vi "Saccade-Analyser.vi"(3 "EMA-Data IN":T4={"Impulse Positions"=[], "No. Imp"=0, "Parameter Time Series"=[], "Parameter Impuls Series"=[], "Experiment Parameters"={"Freq"=0.0, "Vel"=0, "Acc"=0, "Stimulus"=""}, "Autosort File"=refnum, "Data File"={"Data Channels"=[], "Sample Rate"=0, "Channel List"=[]}, "Experiment data path"=path "/Macintosh HD/Users/patrick/Studium/Diploma Thesis/Data Analysis", "Image data path"=path "/Macintosh HD/Users/patrick/Studium/Diploma Thesis/Data Analysis", "LVS data path"=path "/Macintosh HD/Users/patrick/Studium/Diploma Thesis/Data Analysis", "Raw copy path"=path "/Macintosh HD/Users/patrick/Studium/Diploma Thesis/Data Analysis", "filename"="No file selected", "desaccading parameters"={"Tolerance"=0, "Acc Range"=0.0, "Sample Rate"=0, "Impulse Plane 2"=enum."Other", "Impulse dir"=FALSE}, "Experiment Parameters 2"={"Subject"="", "Strain"="", "Rotation plane"="", "Experimenter"="", "Trial"=0.0, "Time"=0.0}, "Excel"={"Excel._Application"=refnum, "Use Excel"=FALSE, "Worksheet SINE"=refnum, "Row SINE"=0, "Worksheet TRANS"=refnum, "Row TRANS"=0}, "Session Config File"=refnum, "Autosort Parameter Set"=1, "EMA Version"="", "desacc "={"Threshold 1 [Acc]"=1617.080808080808, "Threshold 2 [% of TH1]"=67, "tolerance"=5, "Search WD "=0.19090909090909092, " always use TH2"=TRUE, "Range"=3.2323232323232323, "Max time"=200.0, "Min time"=20.0, "Velocity Threshold"=67}, "Cycle Nr for Saccades"={"POS"=0, "NEG"=0}, "calibration name"="No file selected"} {"Parameter Time Series"."time offset" format="%.3f"; "Parameter Time Series"."Gain" format="%.1f"; "Parameter Time Series"."Offset" format="%.1f"; "Parameter Time Series"."List 1" items=["Motor-Pos", "Motor-Vel", "Lx Position-in-Head", "Ly Position-in-Head", "Lz Position-in-Head", "Lx Velocity-in-Head", "Ly Velocity-in-Head", "Lz Velocity-in-Head", "Ll Velocity-in-Head", "Lr Velocity-in-Head", "Lx Accel-in-Head", "Ly Accel-in-Head", "Lz Accel-in-Head", "Rx Position-in-Head", "Ry Position-in-Head", "Rz Position-in-Head", "Rx Velocity-in-Head", "Ry Velocity-in-Head", "Rz Velocity-in-Head", "Rl Velocity-in-Head", "Rr Velocity-in-Head", "Rx Accel-in-Head", "Ry Accel-in-Head", "Rz Accel-in-Head", "Global Trigger", "", "", ""]; "Parameter Impuls Series"."Gain" format="%.1f"; "Parameter Impuls Series"."Offset" format="%.1f"}) -> ()   [LabVIEW 2016]
uses:
  core/type-defs/TD_Statemachine-Data.ctl
  core/type-defs/TD_Time Series.ctl
  core/type-defs/TD_Impulse Parameter.ctl
  Saccade-Analyzer-TD.ctl
  <vilib>/Utility/miscctls.llb/LVRowAndColumnTypeDef.ctl
  <vilib>/Analysis/baseanly.llb/Mean (DBL).vi
  <vilib>/Analysis/3filter.llb/Savitzky-Golay Filter (DBL).vi
  <vilib>/Analysis/1siggen.llb/Ramp Pattern by Samples.vi
  comm/comm.lvlib
  comm/impulse/impulse functions.lvlib
  <vilib>/Analysis/NI_AALBase.lvlib
  <vilib>/Analysis/NI_AALPro.lvlib
  <vilib>/Analysis/NI_AAL_SigProc.lvlib
  comm/nan operations/nan operations.lvlib
  core/core.lvlib
panel:
  in  "Undo Button":bool
  in  "Amend":bool
  out "Saccade Velocity":dbl[][](graph)
  out "Saccade Position":dbl[][](graph)
  in  "Direction":bool
  in  "Start":bool
  in  "Channel Velocity":u16(ring)=13 items=["Hz Position-in-Head", "Hz Velocity-in-Head", "Hy Position-in-Head", "Hy Velocity-in-Head", "Hx Position-in-Head", "Hx Velocity-in-Head", "Hl Velocity-in-Head", "Hr Velocity-in-Head", "Lx Position-in-Head", "Ly Position-in-Head", "Lz Position-in-Head", "Lx Velocity-in-Head", "Ly Velocity-in-Head", "Lz Velocity-in-Head", "Ll Velocity-in-Head", "Lr Velocity-in-Head", "Rx Position-in-Head", "Ry Position-in-Head", "Rz Position-in-Head", "Rx Velocity-in-Head", "Ry Velocity-in-Head", "Rz Velocity-in-Head", "Rl Velocity-in-Head", "Rr Velocity-in-Head", "Target on/off", "aux input 1", "aux input 2", " ", "", "", "", "Target Hor", "Target Ver", ""]
  in  "Channel Position":u16(ring)=13 items=["Hz Position-in-Head", "Hz Velocity-in-Head", "Hy Position-in-Head", "Hy Velocity-in-Head", "Hx Position-in-Head", "Hx Velocity-in-Head", "Hl Velocity-in-Head", "Hr Velocity-in-Head", "Lx Position-in-Head", "Ly Position-in-Head", "Lz Position-in-Head", "Lx Velocity-in-Head", "Ly Velocity-in-Head", "Lz Velocity-in-Head", "Ll Velocity-in-Head", "Lr Velocity-in-Head", "Rx Position-in-Head", "Ry Position-in-Head", "Rz Position-in-Head", "Rx Velocity-in-Head", "Ry Velocity-in-Head", "Rz Velocity-in-Head", "Rl Velocity-in-Head", "Rr Velocity-in-Head", "Target on/off", "aux input 1", "aux input 2", " ", "", "", "", "Target Hor", "Target Ver", ""]
  in  "Tab Control":T1(tab)
  out "Main Sequence - Velocity vs Position":T2(graph)
  out "Saccade Duration":dbl[][](graph)
  in  "Copy to Clipboard":bool
  out "Mean Saccade Duration [ms]":dbl format="%0.2f"
  out "Main Sequence - Duration vs Position":T2(graph)
  in  "Adjust":bool
  in  "Skip for Analysis":bool caption="Cancel Button"
  out "Single Saccade Display":T3(graph)
  in  "Skip Forward Button":bool
  in  "Pause Button":bool
  in  "Seek Forward Button":bool
  out "Mean Noise":dbl
  out "SD Noise":dbl
  in  "Copy to Clipboard 2":bool
  in  "Table":string[][](table)
  # "Saccade / Quick-Phase Analyser"
  # "(c) Patrick Huebner 2011"
  # "POS"
  # "NEG"
  # "+/-"
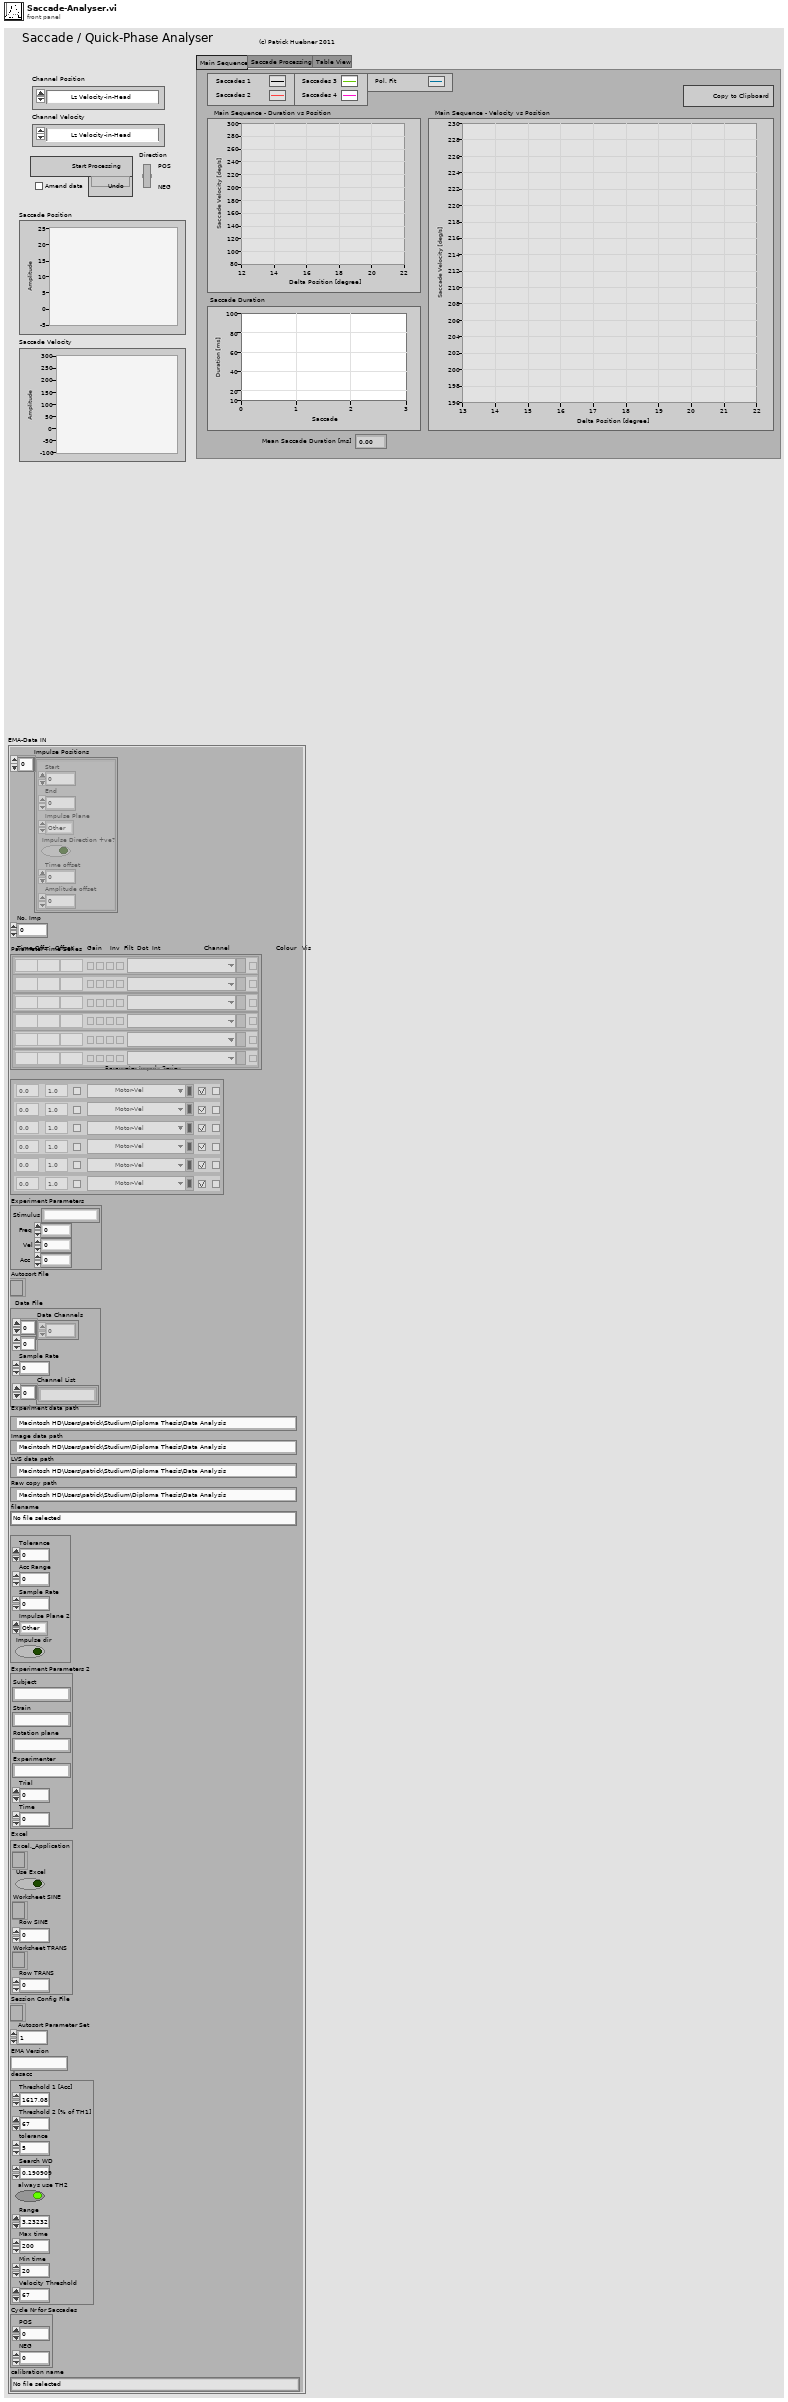
[diagram p1: front panel]
types:
  T1 = enum32{"Main Sequence", "Saccade Processing", "Table View"}
  T2 = cluster{"Best Polynomial Fit":dbl[], "Sorted array":dbl[]}[]
  T3 = cluster{"Ramp Pattern":dbl[], "appended array":dbl[]}[]
  T4 = typedef "core.lvlib/TD_Statemachine-Data.ctl" = cluster{"Impulse Positions":cluster{"Start":i32, "End":i32, "Impulse Plane":enum16{"Other", "Yaw", "Pitch", "Roll", "LARP", "RALP"}, "Impulse Direction +ve?":bool, "Time offset":i32, "Amplitude offset":dbl}[], "No. Imp":i32, "Parameter Time Series":T5, "Parameter Impuls Series":T6, "Experiment Parameters":cluster{"Freq":dbl, "Vel":i32, "Acc":i32, "Stimulus":string}, "Autosort File":refnum<file>, "Data File":cluster{"Data Channels":dbl[][], "Sample Rate":i32, "Channel List":string[]}, "Experiment data path":path, "Image data path":path, "LVS data path":path, "Raw copy path":path, "filename":string, "desaccading parameters":cluster{"Tolerance":i32, "Acc Range":dbl, "Sample Rate":i32, "Impulse Plane 2":enum16{"Other", "Yaw", "Pitch", "Roll", "LARP", "RALP"}, "Impulse dir":bool}, "Experiment Parameters 2":cluster{"Subject":string, "Strain":string, "Rotation plane":string, "Experimenter":string, "Trial":dbl, "Time":dbl}, "Excel":cluster{"Excel._Application":refnum<k7>, "Use Excel":bool, "Worksheet SINE":refnum<k7>, "Row SINE":i32, "Worksheet TRANS":refnum<k7>, "Row TRANS":i32}, "Session Config File":refnum<file>, "Autosort Parameter Set":i32, "EMA Version":string, "desacc ":cluster{"Threshold 1 [Acc]":dbl, "Threshold 2 [% of TH1]":i32, "tolerance":i32, "Search WD ":dbl, " always use TH2":bool, "Range":dbl, "Max time":dbl, "Min time":dbl, "Velocity Threshold":i32}, "Cycle Nr for Saccades":cluster{"POS":i32, "NEG":i32}, "calibration name":string}
  T5 = typedef "core.lvlib/TD_Time Series.ctl" = cluster{"time offset":dbl, "Offset":dbl, "Gain":dbl, "inverse":bool, "filter data":bool, "dots":bool, "interpolate":bool, "List 1":u16, "Color Box":u32, "Boolean":bool}[]
  T6 = typedef "core.lvlib/TD_Impulse Parameter.ctl" = cluster{"Color":u32, "Visible":bool, "Channel":u16, "Invert":bool, "Desaccade":bool, "Offset":dbl, "Gain":dbl}[]
  T7 = typedef "Saccade-Analyzer-TD.ctl" = cluster{"Direction Plot":bool, "Position":dbl[][], "Velocity":dbl[][], "Saccade Counter":i32, "Single Velocity":dbl[], "Single Position":dbl[], "Single Acceleration":dbl[], "Saccade Onset":cluster{"X":dbl, "Y":dbl}, "Linear Fit":dbl[], "Saccade End":cluster{"X":dbl, "Y":dbl}, "Acceleration Peak":i32, "Amendments":i32, "Duration":cluster{"Duration":dbl[]}[], "Peak Velocity":cluster{"Duration":dbl[]}[], "Position Difference":cluster{"Duration":dbl[]}[], "EYE":string[], "Direction":bool[], "Table1 size":i32, "Mean Noise":dbl, "SD Noise":dbl}
  T8 = typedef "LVRowAndColumnTypeDef.ctl" = cluster{"Row":i32, "Column":i32}
  T9 = cluster{"Sorted array":dbl[], "Best Polynomial Fit":dbl[]}
  T10 = cluster{"Sorted array":dbl[], "Best Polynomial Fit":dbl[]}[]
  T11 = cluster{"Data Channels":dbl[][], "Sample Rate":i32, "Channel List":string[]}
  T12 = cluster{"Start":i32, "End":i32, "Impulse Plane":enum16{"Other", "Yaw", "Pitch", "Roll", "LARP", "RALP"}, "Impulse Direction +ve?":bool, "Time offset":i32, "Amplitude offset":dbl}[]
  T13 = enum16{"Other", "Yaw", "Pitch", "Roll", "LARP", "RALP"}
  T14 = cluster{"Color":u32, "Visible":bool, "Channel":u16, "Invert":bool, "Desaccade":bool, "Offset":dbl, "Gain":dbl}
  T15 = cluster{"Color":u32, "Visible":bool, "Channel":u16, "Invert":bool, "Desaccade":bool, "Offset":dbl, "Gain":dbl}[]
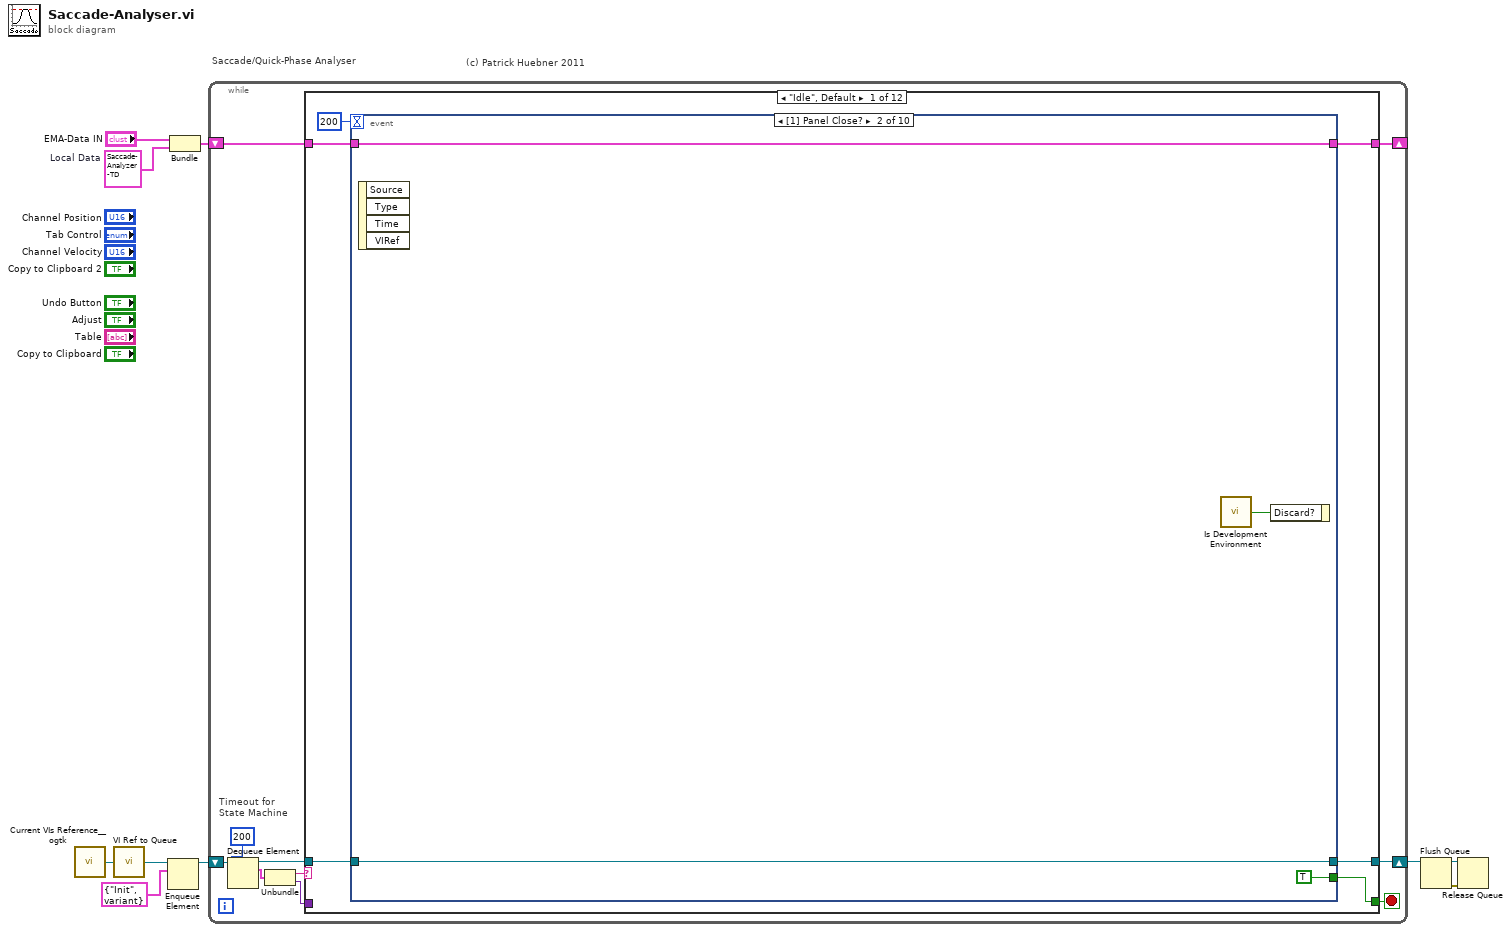
[diagram p0: block diagram]
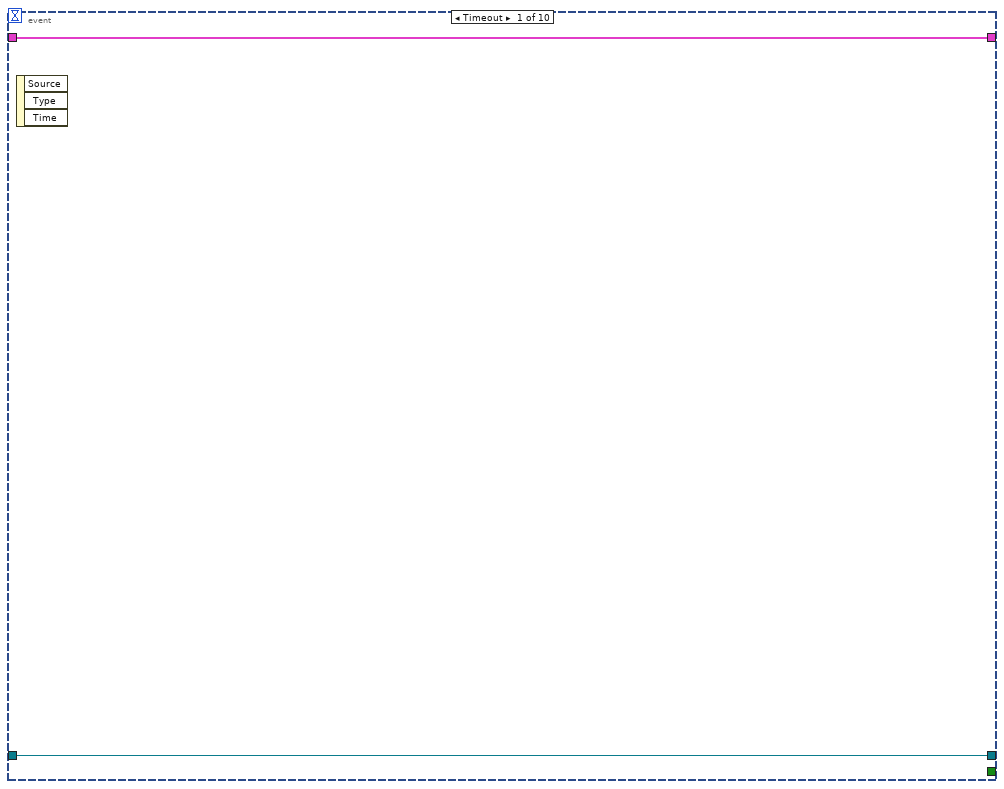
[diagram p2: hidden frame]
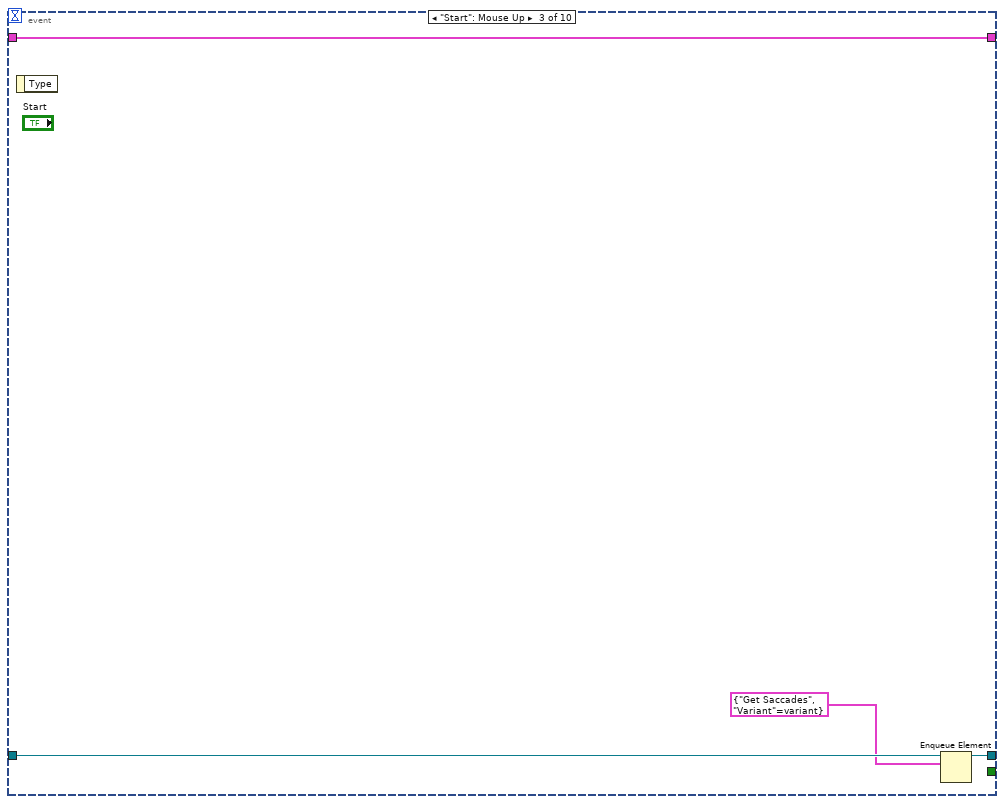
[diagram p3: hidden frame]
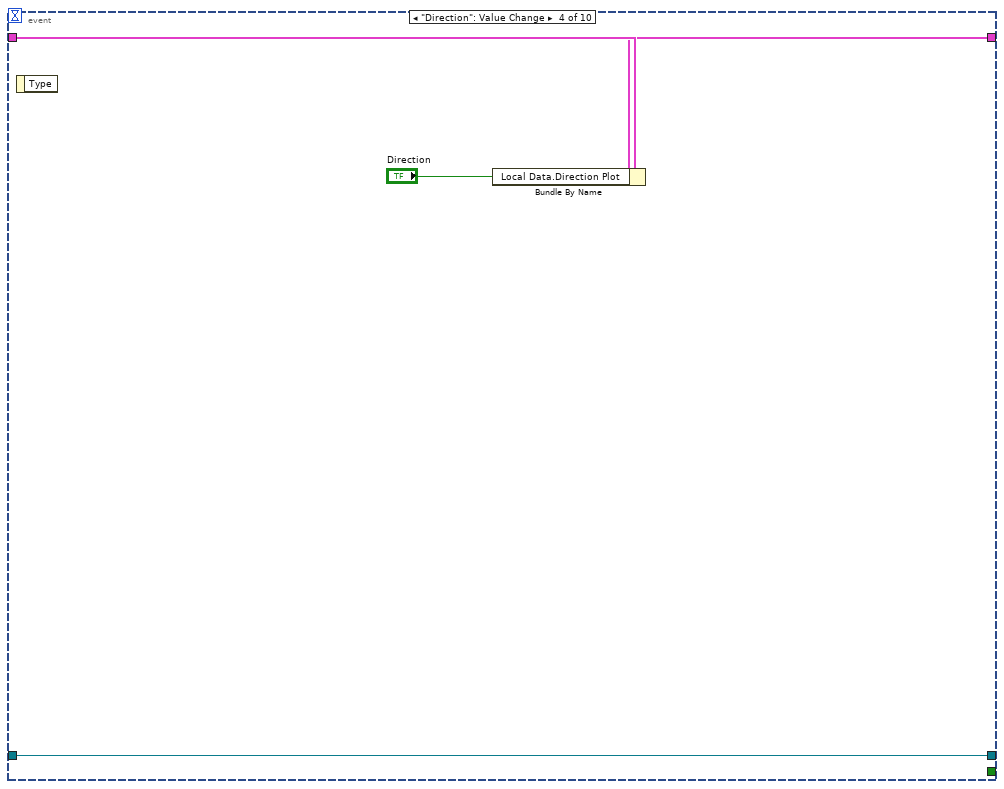
[diagram p4: hidden frame]
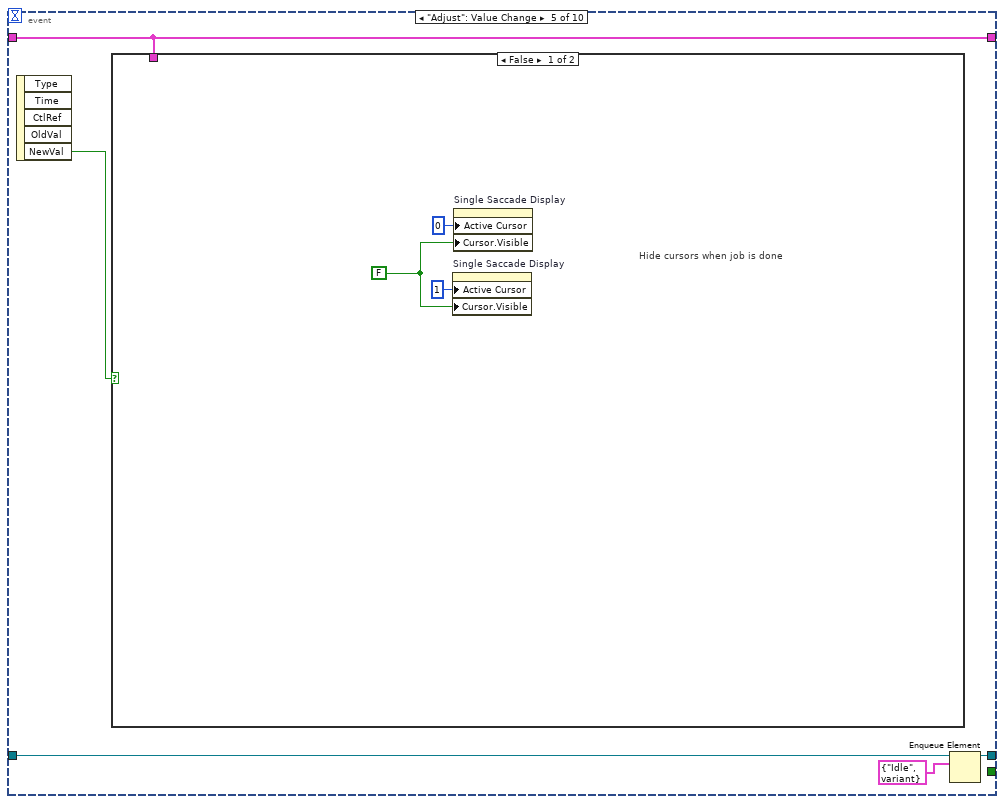
[diagram p5: hidden frame]
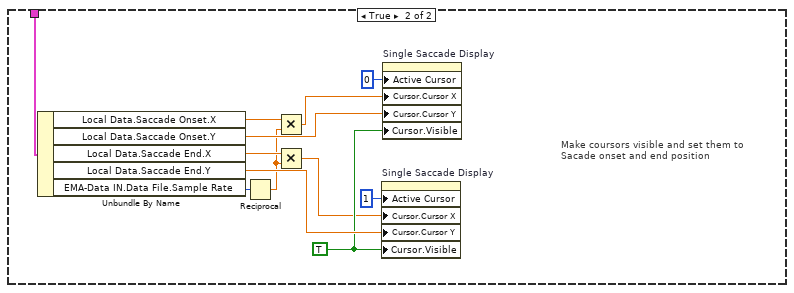
[diagram p6: hidden frame]
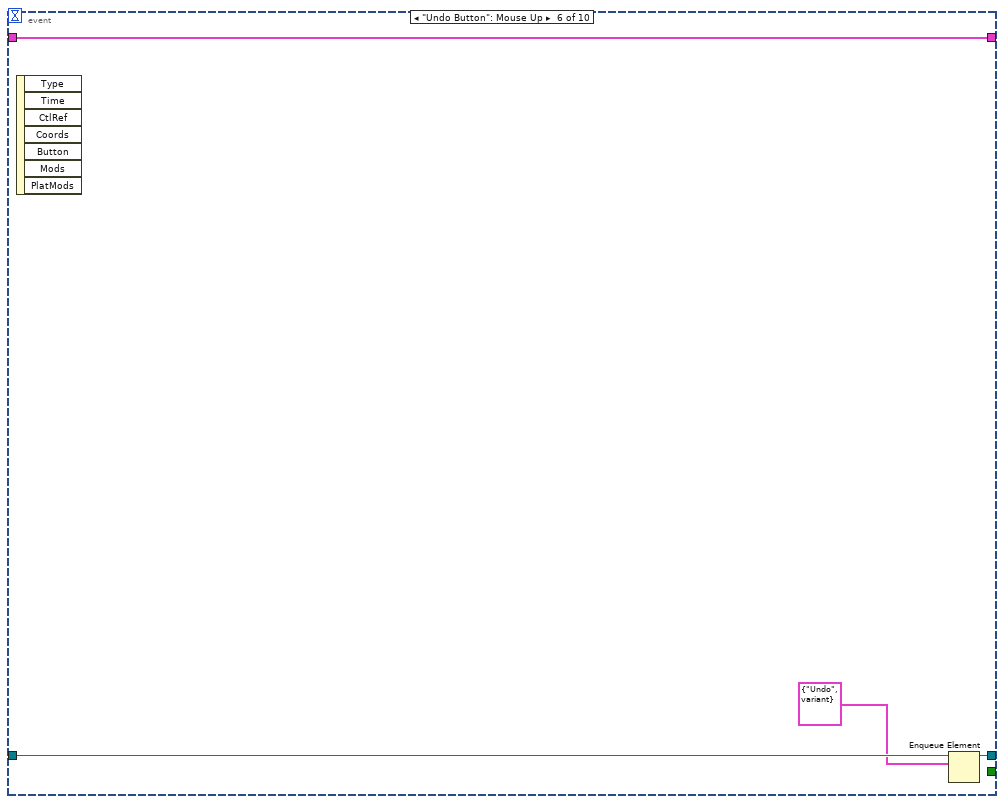
[diagram p7: hidden frame]
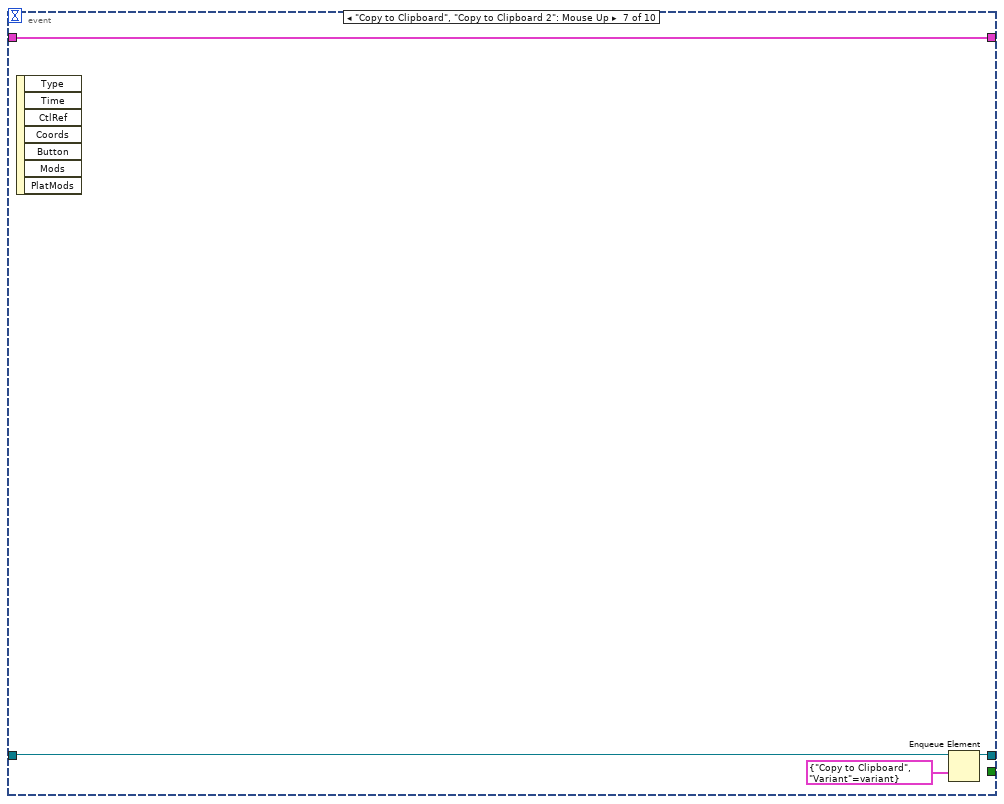
[diagram p8: hidden frame]
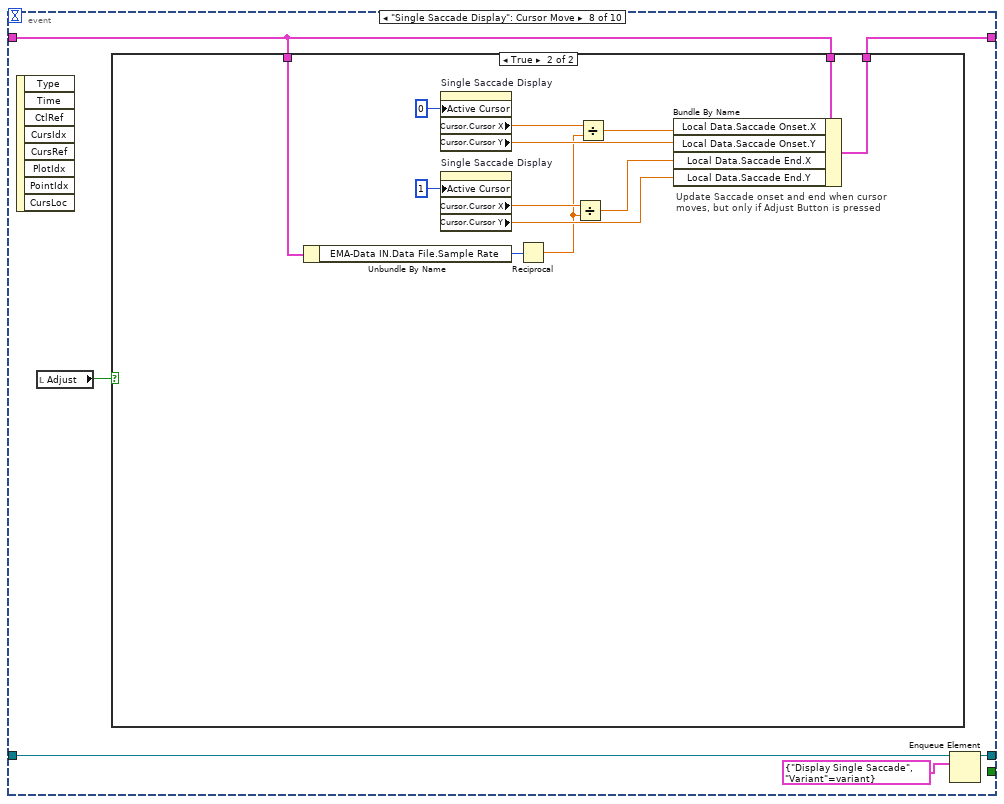
[diagram p9: hidden frame]
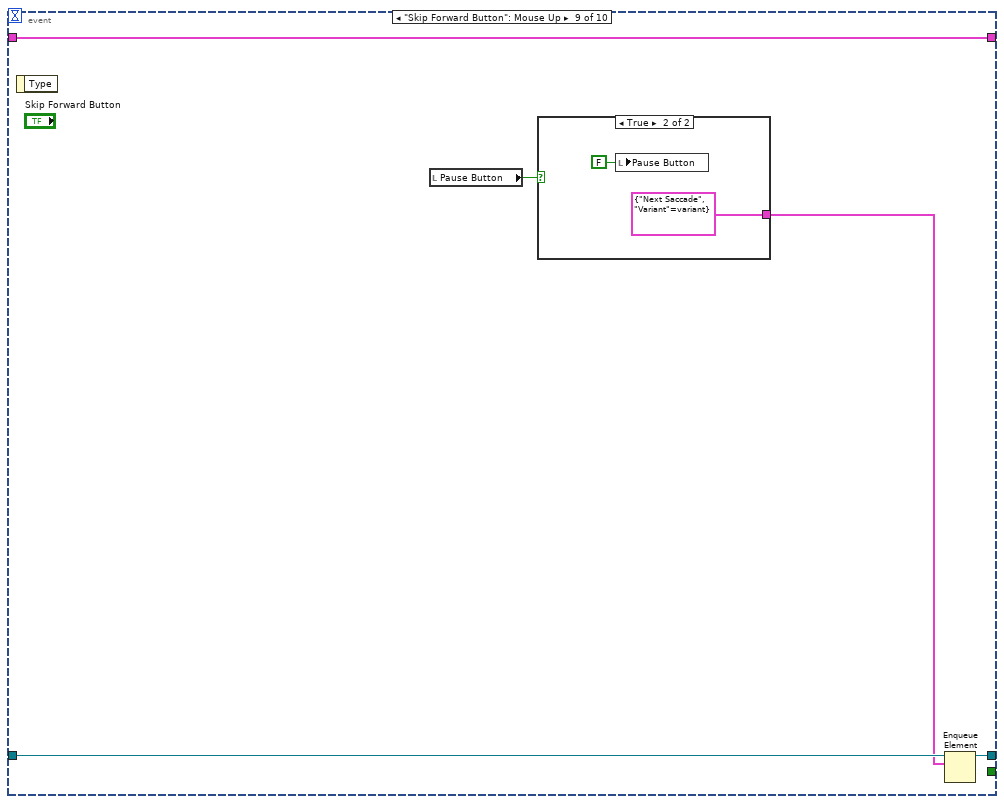
[diagram p11: hidden frame]
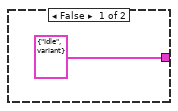
[diagram p12: hidden frame]
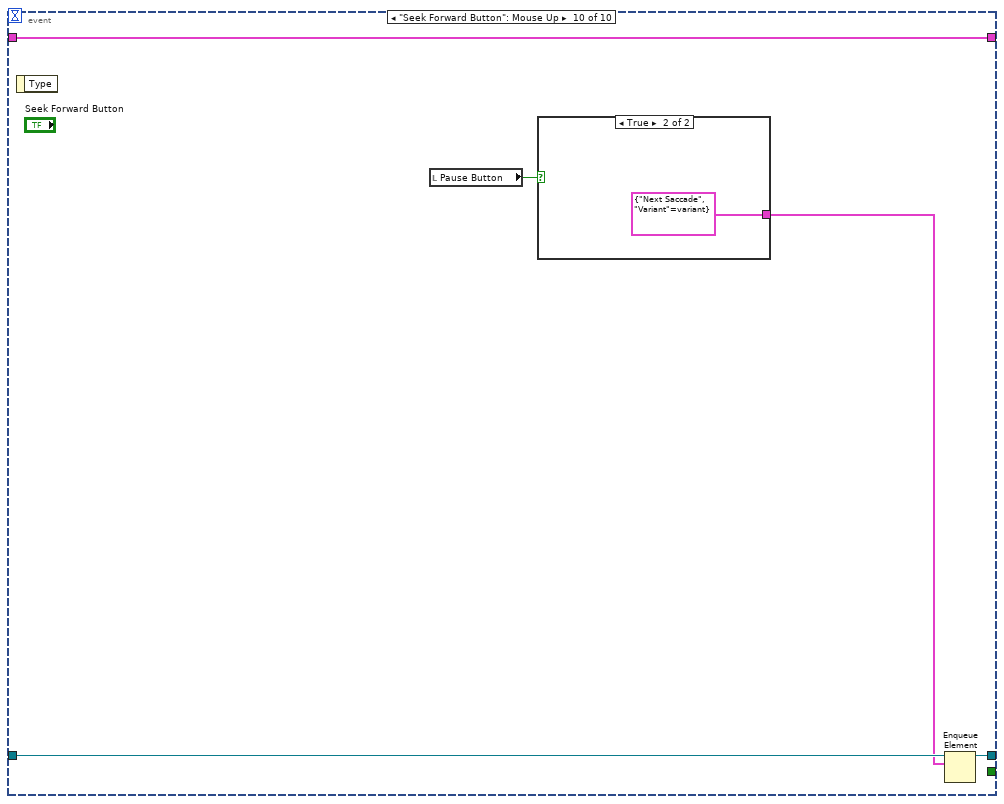
[diagram p13: hidden frame]
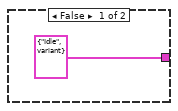
[diagram p14: hidden frame]
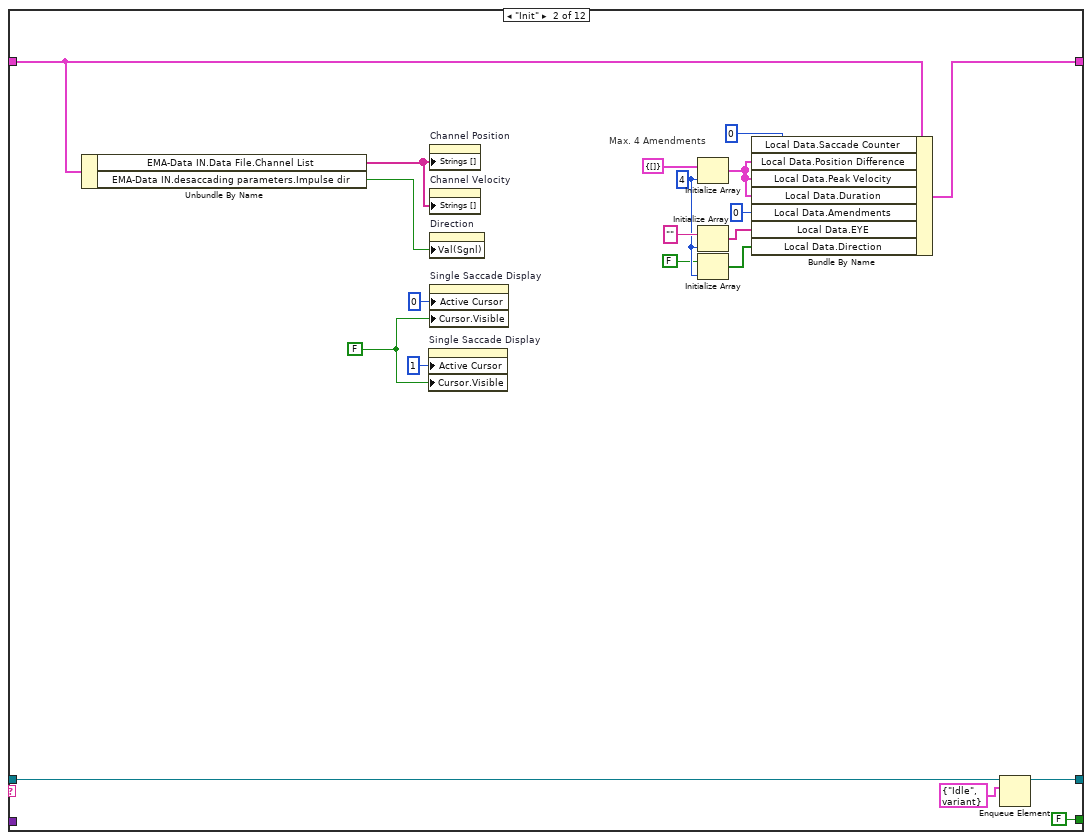
[diagram p15: hidden frame]
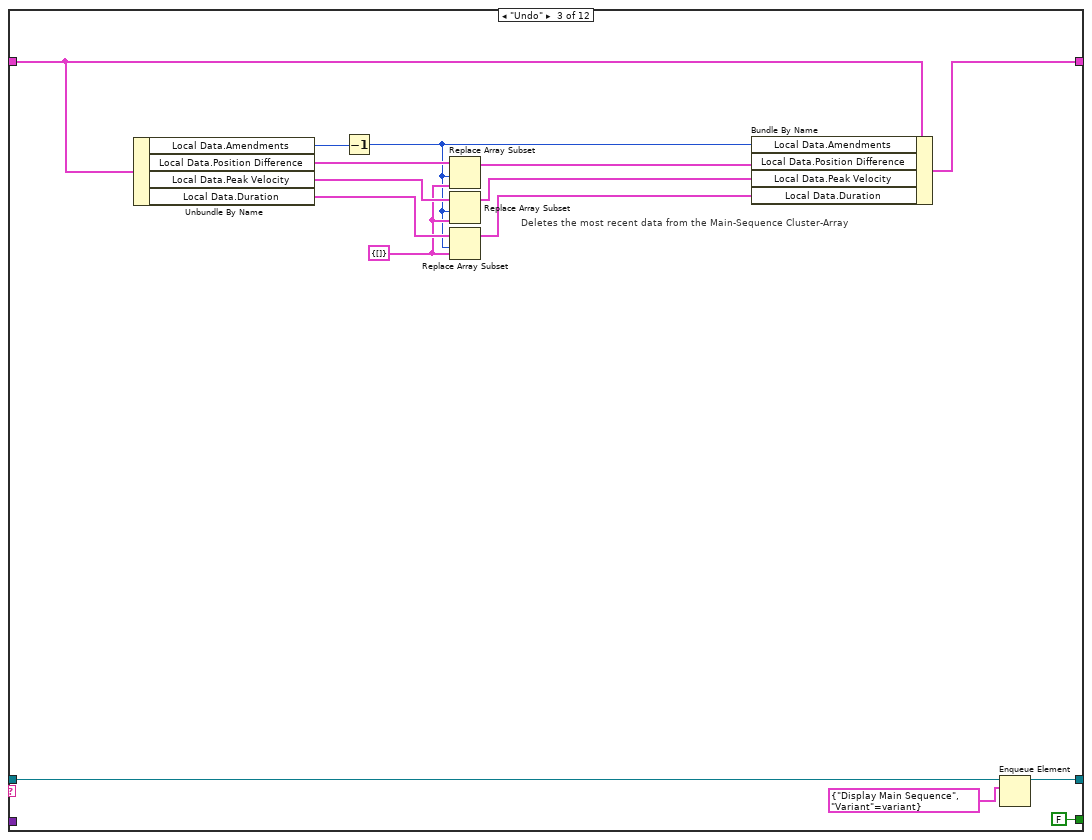
[diagram p16: hidden frame]
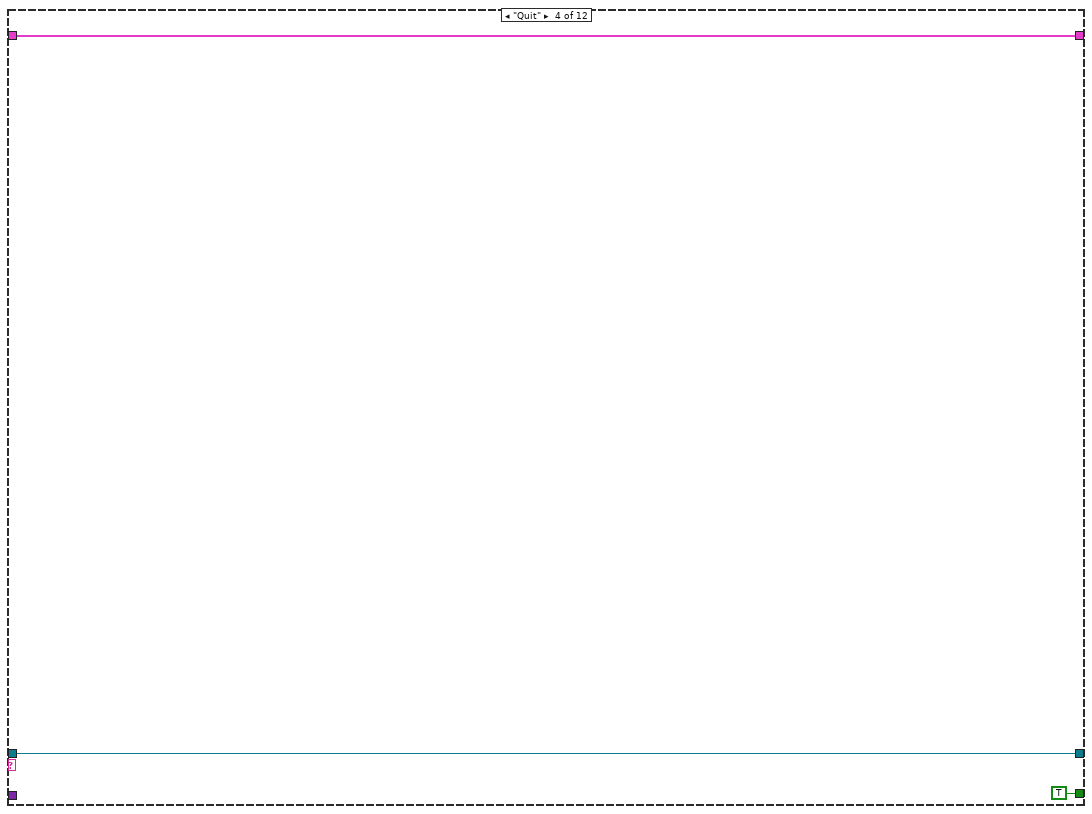
[diagram p17: hidden frame]
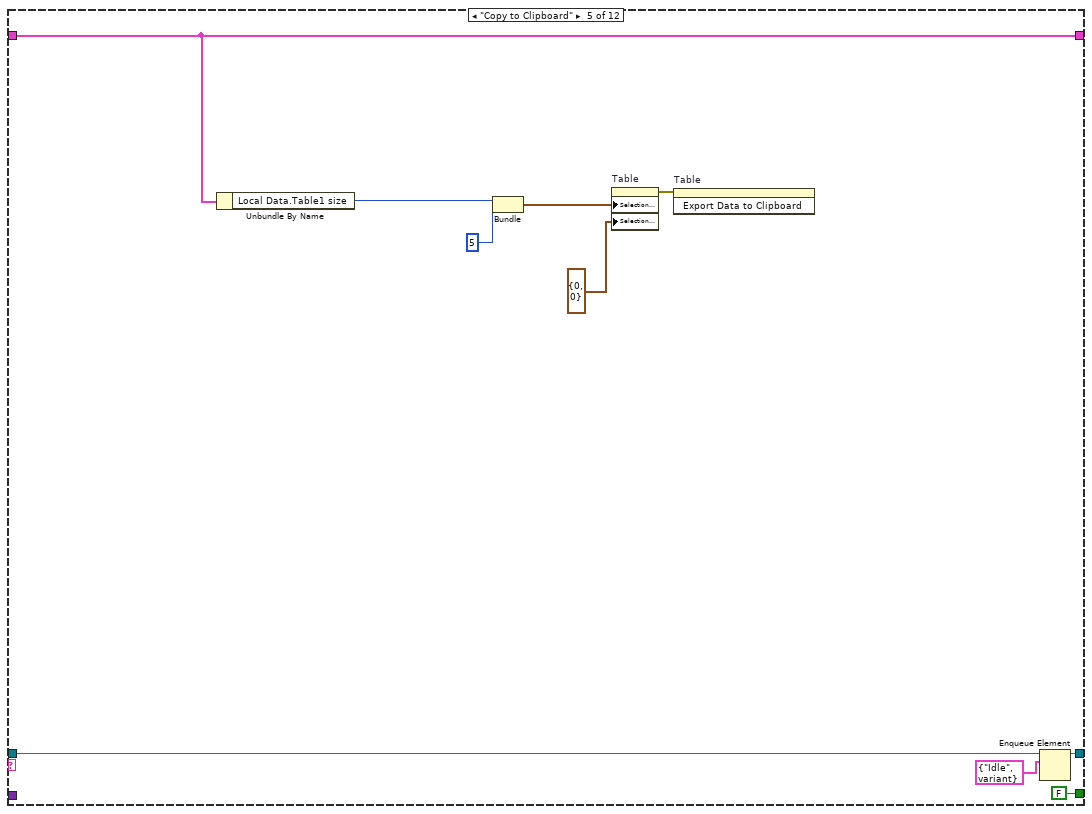
[diagram p18: hidden frame]
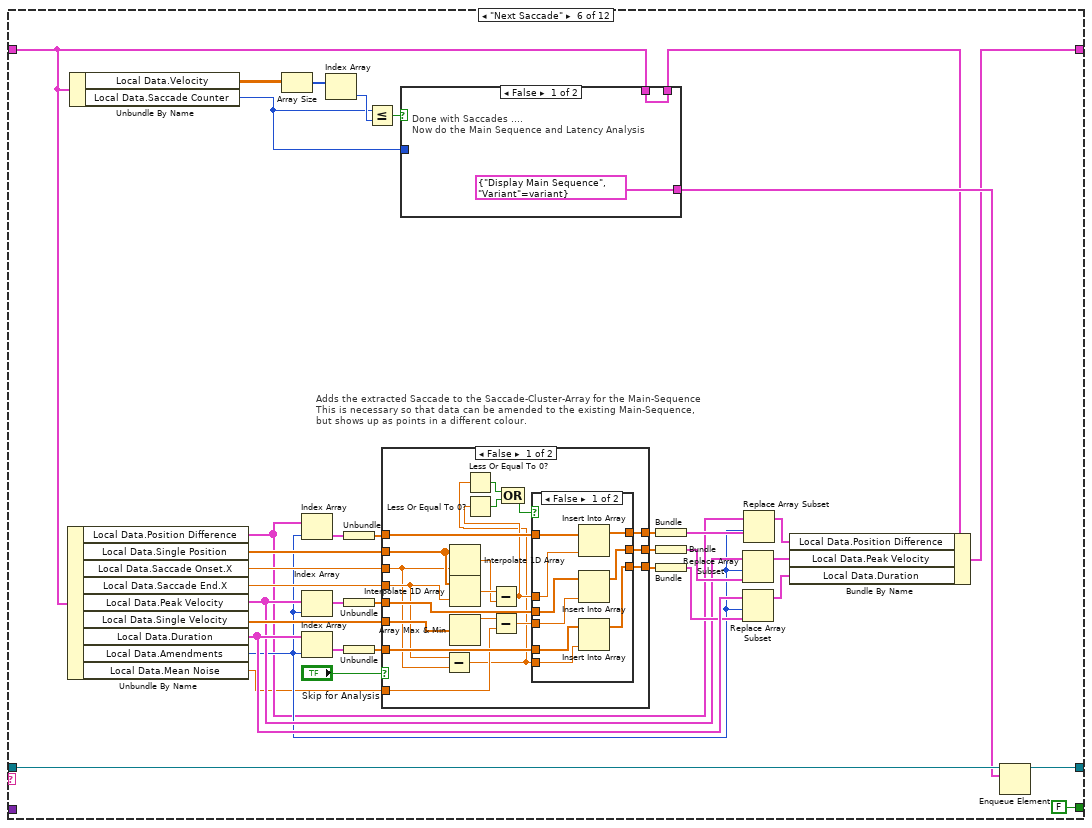
[diagram p19: hidden frame]
diagram:
  w1 = T7 {"Direction Plot"=FALSE, "Position"=[], "Velocity"=[], "Saccade Counter"=0, "Single Velocity"=[], "Single Position"=[], "Single Acceleration"=[], "Saccade Onset"={"X"=0.0, "Y"=0.0}, "Linear Fit"=[], "Saccade End"={"X"=0.0, "Y"=0.0}, "Acceleration Peak"=0, "Amendments"=0, "Duration"=[], "Peak Velocity"=[], "Position Difference"=[], "EYE"=[], "Direction"=[], "Table1 size"=0, "Mean Noise"=0.0, "SD Noise"=0.0}  # Local Data
  # "(c) Patrick Huebner 2011"
  # "Saccade/Quick-Phase Analyser"
  n1 = call <userlib>:"Current VIs Reference__ogtk.vi"() -> ("Current VI's reference"=w8:refnum<vi>)  [unwired: 5 in]
  n2 = call "VI Ref to Queue.vi"("VI Refnum"=w8) -> ("queue out"=w9:refnum<queue>)  [unwired: 4 in]
  n3 = Enqueue Element(queue=w9, element=cluster{string, "Variant":variant} {"Init", "Variant"=variant}) -> (queue out=w7:refnum<queue>)  [unwired: 2 in, 2 out]
  n4 = Bundle("EMA-Data IN"="EMA-Data IN", "Local Data"=w1) -> (w3:cluster{"EMA-Data IN":T4, "Local Data":T7})  [unwired: 1 in]
  n5 = while {
    shift-right: [w15] -> w4
    shift-left: w7 -> [w19]
    shift-right: [w11] -> _
    shift-left: w3 -> [w12]
    stop <- w14 stop-if-true
    # "Timeout for \nState Machine"
    n6 = Dequeue Element(queue=w19, timeout in ms (-1)=200) -> (queue out=w16:refnum<queue>, element=w20:cluster{string, "Variant":variant})  [unwired: 1 in, 2 out]
    n7 = Unbundle(w20) -> (w18:string, "Variant"=w17:variant)
    n8 = case shown="\"Idle\", Default" w18 {
      tunnel: w17 -> [_ _ _ _ _ _ _ _ _ _ _ _]
      tunnel: w16 -> [w26 w121 w136 w139 w149 w186 w281 w327 w400 w526 w574 w612]
      tunnel: [w25 w122 w137 w139 w150 w187 w282 w328 w401 w527 w575 w613] -> w15
      tunnel: [w21 FALSE FALSE TRUE FALSE FALSE _ w329 FALSE FALSE FALSE FALSE] -> w14
      tunnel: w12 -> [w23 w117 w134 w140 w143 w179 w261 w305 w393 w524 w573 w586]
      tunnel: [w22 w116 w133 w140 w143 w175 w260 w304 w392 w523 w573 w597] -> w11
      frame "Idle", Default {
        n9 = event shown="[1] Panel Close?" {
          selector: _ -> [_ _ _ _ _ _ _ _ _ _]
          dyn-events: _ -> [_ _ _ _ _ _ _ _ _ _]
          timeout: 200 -> [_ _ _ _ _ _ _ _ _ _]
          tunnel: w26 -> [w27 w32 w34 w38 w42 w62 w67 w73 w91 w99]
          tunnel: [w27 w32 w35 w38 w43 w63 w68 w74 w92 w100] -> w25
          tunnel: w23 -> [w28 w31 w36 w40 w44 w64 w65 w69 w89 w97]
          tunnel: [w28 w31 w36 w39 w44 w64 w65 w71 w89 w97] -> w22
          tunnel: [_ TRUE _ _ _ _ _ _ _ _] -> w21
          event Timeout {
            n10 = event-data() -> ()  [unwired: 1 in, 3 out]
          }
          event Panel Close? {
            n11 = event-data() -> ()  [unwired: 1 in, 4 out]
            n12 = call <userlib>:"Is Development Environment.vi"() -> ("exe?"=w30:bool)  [unwired: 5 in]
            n13 = event-data("Discard?"=w30) -> ()  [unwired: 1 in, 1 out]
          }
          event "Start": Mouse Up {
            n14 = event-data() -> ()  [unwired: 1 in, 1 out]
            n15 = Enqueue Element(queue=w34, element=cluster{string, "Variant":variant} {"Get Saccades", "Variant"=variant}) -> (queue out=w35:refnum<queue>)  [unwired: 2 in, 2 out]
          }
          event "Direction": Value Change {
            n16 = event-data() -> ()  [unwired: 1 in, 1 out]
            n17 = Bundle By Name(cluster=w40, "Local Data.Direction Plot"="Direction") -> (w39:cluster{"EMA-Data IN":T4, "Local Data":T7})
          }
          event "Adjust": Value Change {
            n18 = event-data() -> ("NewVal"=w45:bool)  [unwired: 1 in, 4 out]
            n19 = case shown="False" w45 {
              tunnel: w44 -> [_ w58]
              frame False {
                w46 = FALSE ("Cursor.Visible")
                # "Hide cursors when job is done"
                n20 = property on="Single Saccade Display" class="XYGraph (strict)"("Active Cursor"=u32 1, "Cursor.Visible"=w46) -> ()  [unwired: 2 in, 2 out]
                n21 = property on="Single Saccade Display" class="XYGraph (strict)"("Active Cursor"=u32 0, "Cursor.Visible"=w46) -> ()  [unwired: 2 in, 2 out]
              }
              frame True {
                w53 = TRUE ("Cursor.Visible")
                # "Make coursors visible and set them to\nSacade onset and end position"
                n22 = Unbundle By Name(w58) -> ("Local Data.Saccade Onset.X"=w57:dbl, "Local Data.Saccade Onset.Y"=w56:dbl, "Local Data.Saccade End.X"=w55:dbl, "Local Data.Saccade End.Y"=w54:dbl, "EMA-Data IN.Data File.Sample Rate"=w52:i32)
                n23 = Reciprocal(x=w52) -> (1/x=w49:dbl)
                n24 = Multiply(x=w57, y=w49) -> (x*y=w51:dbl)
                n25 = Multiply(x=w55, y=w49) -> (x*y=w50:dbl)
                n26 = property on="Single Saccade Display" class="XYGraph (strict)"("Active Cursor"=u32 1, "Cursor.Cursor X"=w50, "Cursor.Cursor Y"=w54, "Cursor.Visible"=w53) -> ()  [unwired: 2 in, 2 out]
                n27 = property on="Single Saccade Display" class="XYGraph (strict)"("Active Cursor"=u32 0, "Cursor.Cursor X"=w51, "Cursor.Cursor Y"=w56, "Cursor.Visible"=w53) -> ()  [unwired: 2 in, 2 out]
              }
            }
            n28 = Enqueue Element(queue=w42, element=cluster{string, "Variant":variant} {"Idle", "Variant"=variant}) -> (queue out=w43:refnum<queue>)  [unwired: 2 in, 2 out]
          }
          event "Undo Button": Mouse Up {
            n29 = event-data() -> ()  [unwired: 1 in, 7 out]
            n30 = Enqueue Element(queue=w62, element=cluster{string, "Variant":variant} {"Undo", "Variant"=variant}) -> (queue out=w63:refnum<queue>)  [unwired: 2 in, 2 out]
          }
          event "Copy to Clipboard", "Copy to Clipboard 2": Mouse Up {
            n31 = event-data() -> ()  [unwired: 1 in, 7 out]
            n32 = Enqueue Element(queue=w67, element=cluster{string, "Variant":variant} {"Copy to Clipboard", "Variant"=variant}) -> (queue out=w68:refnum<queue>)  [unwired: 2 in, 2 out]
          }
          event "Single Saccade Display": Cursor Move {
            n33 = event-data() -> ()  [unwired: 1 in, 8 out]
            n34 = local read "Adjust"() -> (w70:bool)
            n35 = case shown="True" w70 {
              tunnel: w69 -> [w75 w86]
              tunnel: [w75 w85] -> w71
              tunnel: w69 -> [_ w80]
              frame False {
              }
              frame True {
                # "Update Saccade onset and end when cursor moves, but only if Adjust Button is pressed"
                n36 = Unbundle By Name(w80) -> ("EMA-Data IN.Data File.Sample Rate"=w79:i32)
                n37 = property on="Single Saccade Display" class="XYGraph (strict)"("Active Cursor"=u32 0) -> ("Cursor.Cursor X"=w84:dbl, "Cursor.Cursor Y"=w83:dbl)  [unwired: 2 in, 2 out]
                n38 = property on="Single Saccade Display" class="XYGraph (strict)"("Active Cursor"=u32 1) -> ("Cursor.Cursor X"=w82:dbl, "Cursor.Cursor Y"=w81:dbl)  [unwired: 2 in, 2 out]
                n39 = Reciprocal(x=w79) -> (1/x=w76:dbl)
                n40 = Divide(x=w82, y=w76) -> (x/y=w78:dbl)
                n41 = Divide(x=w84, y=w76) -> (x/y=w77:dbl)
                n42 = Bundle By Name(cluster=w86, "Local Data.Saccade Onset.X"=w77, "Local Data.Saccade Onset.Y"=w83, "Local Data.Saccade End.X"=w78, "Local Data.Saccade End.Y"=w81) -> (w85:cluster{"EMA-Data IN":T4, "Local Data":T7})
              }
            }
            n43 = Enqueue Element(queue=w73, element=cluster{string, "Variant":variant} {"Display Single Saccade", "Variant"=variant}) -> (queue out=w74:refnum<queue>)  [unwired: 2 in, 2 out]
          }
          event "Skip Forward Button": Mouse Up {
            n44 = event-data() -> ()  [unwired: 1 in, 1 out]
            n45 = local read "Pause Button"() -> (w93:bool)
            n46 = case shown="True" w93 {
              tunnel: [cluster{string, "Variant":variant} {"Idle", "Variant"=variant} ("element") cluster{string, "Variant":variant} {"Next Saccade", "Variant"=variant} ("element")] -> w90
              frame False {
              }
              frame True {
                n47 = local write "Pause Button"(FALSE ("Pause Button")) -> ()
              }
            }
            n48 = Enqueue Element(queue=w91, element=w90) -> (queue out=w92:refnum<queue>)  [unwired: 2 in, 2 out]
          }
          event "Seek Forward Button": Mouse Up {
            n49 = event-data() -> ()  [unwired: 1 in, 1 out]
            n50 = local read "Pause Button"() -> (w101:bool)
            n51 = case shown="True" w101 {
              tunnel: [cluster{string, "Variant":variant} {"Idle", "Variant"=variant} ("element") cluster{string, "Variant":variant} {"Next Saccade", "Variant"=variant} ("element")] -> w98
              frame False {
              }
              frame True {
              }
            }
            n52 = Enqueue Element(queue=w99, element=w98) -> (queue out=w100:refnum<queue>)  [unwired: 2 in, 2 out]
          }
        }
      }
      frame "Init" {
        w109 = FALSE ("Cursor.Visible")
        w105 = 4 ("dimension size")
        # "Max. 4 Amendments"
        n53 = Unbundle By Name(w117) -> ("EMA-Data IN.Data File.Channel List"=w119:string[], "EMA-Data IN.desaccading parameters.Impulse dir"=w118:bool)
        n54 = property on="Single Saccade Display" class="XYGraph (strict)"("Active Cursor"=u32 1, "Cursor.Visible"=w109) -> ()  [unwired: 2 in, 2 out]
        n55 = property on="Channel Position" class="Ring (strict)"("Strings []"=w119) -> ()  [unwired: 2 in, 2 out]
        n56 = property on="Channel Velocity" class="Ring (strict)"("Strings []"=w119) -> ()  [unwired: 2 in, 2 out]
        n57 = property on="Direction" class="Bool (strict)"("Val(Sgnl)"=w118) -> ()  [unwired: 2 in, 2 out]
        n58 = property on="Single Saccade Display" class="XYGraph (strict)"("Active Cursor"=u32 0, "Cursor.Visible"=w109) -> ()  [unwired: 2 in, 2 out]
        n59 = Initialize Array(cluster{"Duration":dbl[]} {"Duration"=[]} ("Cluster"), w105) -> (w112:cluster{"Duration":dbl[]}[])
        n60 = Initialize Array("" ("String"), w105) -> (w107:string[])
        n61 = Initialize Array(FALSE, w105) -> (w106:bool[])
        n62 = Bundle By Name(cluster=w117, "Local Data.Saccade Counter"=0, "Local Data.Position Difference"=w112, "Local Data.Peak Velocity"=w112, "Local Data.Duration"=w112, "Local Data.Amendments"=0, "Local Data.EYE"=w107, "Local Data.Direction"=w106) -> (w116:cluster{"EMA-Data IN":T4, "Local Data":T7})
        n63 = Enqueue Element(queue=w121, element=cluster{string, "Variant":variant} {"Idle", "Variant"=variant}) -> (queue out=w122:refnum<queue>)  [unwired: 2 in, 2 out]
      }
      frame "Undo" {
        w128 = cluster{"Duration":dbl[]} {"Duration"=[]} ("Cluster")
        # "Deletes the most recent data from the Main-Sequence Cluster-Array"
        n64 = Unbundle By Name(w134) -> ("Local Data.Amendments"=w129:i32, "Local Data.Position Difference"=w132:cluster{"Duration":dbl[]}[], "Local Data.Peak Velocity"=w131:cluster{"Duration":dbl[]}[], "Local Data.Duration"=w130:cluster{"Duration":dbl[]}[])
        n65 = Decrement(x=w129) -> (x-1=w124:i32)
        n66 = Replace Array Subset(array=w132, new element=w128, index=w124) -> (w127:cluster{"Duration":dbl[]}[])
        n67 = Replace Array Subset(array=w131, new element=w128, index=w124) -> (w126:cluster{"Duration":dbl[]}[])
        n68 = Replace Array Subset(array=w130, new element=w128, index=w124) -> (w125:cluster{"Duration":dbl[]}[])
        n69 = Bundle By Name(cluster=w134, "Local Data.Amendments"=w124, "Local Data.Position Difference"=w127, "Local Data.Peak Velocity"=w126, "Local Data.Duration"=w125) -> (w133:cluster{"EMA-Data IN":T4, "Local Data":T7})
        n70 = Enqueue Element(queue=w136, element=cluster{string, "Variant":variant} {"Display Main Sequence", "Variant"=variant}) -> (queue out=w137:refnum<queue>)  [unwired: 2 in, 2 out]
      }
      frame "Quit" {
      }
      frame "Copy to Clipboard" {
        n71 = Unbundle By Name(w143) -> ("Local Data.Table1 size"=w142:i32)
        n72 = Bundle("Table1 size"=w142, "Column"=5) -> (w144:cluster{"Table1 size":i32, "Column":i32})  [unwired: 1 in]
        n73 = property on="Table" class="Tbl (strict)"("Selection Size"=w144, "Selection Start"=T8 {"Row"=0, "Column"=0}) -> (error out=w147:errorcluster)  [unwired: 2 in, 1 out]
        n74 = invoke on="Table" class="Tbl (strict)" method="Export Data to Clipboard"(error in=w147) -> ()  [unwired: 2 in, 3 out]
        n75 = Enqueue Element(queue=w149, element=cluster{string, "Variant":variant} {"Idle", "Variant"=variant}) -> (queue out=w150:refnum<queue>)  [unwired: 2 in, 2 out]
      }
      frame "Next Saccade" {
        # "Adds the extracted Saccade to the Saccade-Cluster-Array for the Main-Sequence\nThis is necessary so that data can be amended to the existing Main-Sequence,\nbut shows up as points in a different colour."
        n76 = Unbundle By Name(w179) -> ("Local Data.Position Difference"=w153:cluster{"Duration":dbl[]}[], "Local Data.Single Position"=w178:dbl[], "Local Data.Saccade Onset.X"=w174:dbl, "Local Data.Saccade End.X"=w173:dbl, "Local Data.Peak Velocity"=w155:cluster{"Duration":dbl[]}[], "Local Data.Single Velocity"=w177:dbl[], "Local Data.Duration"=w164:cluster{"Duration":dbl[]}[], "Local Data.Amendments"=w154:i32, "Local Data.Mean Noise"=w152:dbl)
        n77 = Unbundle By Name(w179) -> ("Local Data.Velocity"=w185:dbl[][], "Local Data.Saccade Counter"=w181:i32)
        n78 = Array Size(array=w185) -> (size(s)=w184:i32[])
        n79 = Index Array(array=w153, index=w154) -> (element=w171:cluster{"Duration":dbl[]})
        n80 = Index Array(array=w155, index=w154) -> (element=w170:cluster{"Duration":dbl[]})
        n81 = Index Array(array=w164, index=w154) -> (element=w167:cluster{"Duration":dbl[]})
        n82 = Index Array(array=w184) -> (element=w183:i32)  [unwired: 1 in]
        n83 = Unbundle(w171) -> ("Duration"=w169:dbl[])
        n84 = Unbundle(w170) -> ("Duration"=w168:dbl[])
        n85 = Unbundle(w167) -> ("Duration"=w166:dbl[])
        n86 = Less Or Equal?(x=w181, y=w183) -> (x <= y?=w182:bool)
        n87 = case shown="False" "Skip for Analysis" {
          tunnel: w178 -> [w208 _]
          tunnel: w169 -> [w197 w224]
          tunnel: [w205 w224] -> w160
          tunnel: w177 -> [w204 _]
          tunnel: w168 -> [w203 w223]
          tunnel: w166 -> [w202 w222]
          tunnel: w173 -> [w201 _]
          tunnel: w174 -> [w200 _]
          tunnel: [w199 w223] -> w161
          tunnel: [w198 w222] -> w165
          tunnel: w152 -> [w195 _]
          frame False {
            n88 = Subtract(x=w201, y=w200) -> (x-y=w192:dbl)
            n89 = Interpolate 1D Array(1:w200, 2:w208) -> (0:w206:dbl)
            n90 = Interpolate 1D Array(1:w201, 2:w208) -> (0:w207:dbl)
            n91 = Array Max & Min(array=w204) -> (max value=w196:dbl)  [unwired: 3 out]
            n92 = Less Or Equal To 0?(x=w192) -> (x <= 0?=w191:bool)
            n93 = Subtract(x=w207, y=w206) -> (x-y=w193:dbl)
            n94 = Less Or Equal To 0?(x=w193) -> (x <= 0?=w190:bool)
            n95 = Subtract(x=w196, y=w195) -> (x-y=w194:dbl)
            n96 = Compound Arithmetic op=OR(w191, w190) -> (w189:bool)
            n97 = case shown="False" w189 {
              tunnel: [w217 w220] -> w205
              tunnel: w203 -> [w216 w219]
              tunnel: w202 -> [w215 w218]
              tunnel: w192 -> [w214 _]
              tunnel: [w213 w219] -> w199
              tunnel: [w212 w218] -> w198
              tunnel: w197 -> [w211 w220]
              tunnel: w193 -> [w210 _]
              tunnel: w194 -> [w209 _]
              frame False {
                n98 = Insert Into Array(array=w211, new element=w210) -> (w217:dbl[])  [unwired: 1 in]
                n99 = Insert Into Array(array=w216, new element=w209) -> (w213:dbl[])  [unwired: 1 in]
                n100 = Insert Into Array(array=w215, new element=w214) -> (w212:dbl[])  [unwired: 1 in]
              }
              frame True {
              }
            }
          }
          frame True {
            n101 = local write "Skip for Analysis"(FALSE ("Skip for Analysis")) -> ()
          }
        }
        n102 = case shown="False" w182 {
          tunnel: w181 -> [_ w231]
          tunnel: w179 -> [w226 w230]
          tunnel: [w226 w228] -> w176
          tunnel: [cluster{string, "Variant":variant} {"Display Main Sequence", "Variant"=variant} ("element") cluster{string, "Variant":variant} {"Extract Features 1", "Variant"=variant} ("element")] -> w180
          frame False {
            # "Done with Saccades ....\nNow do the Main Sequence and Latency Analysis"
          }
          frame True {
            # "More Saccades to analyze ..."
            n103 = Increment(x=w231) -> (x+1=w229:i32)
            n104 = Bundle By Name(cluster=w230, "Local Data.Saccade Counter"=w229) -> (w228:cluster{"EMA-Data IN":T4, "Local Data":T7})
          }
        }
        n105 = Bundle("Duration"=w160) -> (w159:cluster{"Duration":dbl[]})  [unwired: 1 in]
        n106 = Bundle("Duration"=w161) -> (w158:cluster{"Duration":dbl[]})  [unwired: 1 in]
        n107 = Bundle("Duration"=w165) -> (w163:cluster{"Duration":dbl[]})  [unwired: 1 in]
        n108 = Replace Array Subset(array=w155, new element=w158, index=w154) -> (w156:cluster{"Duration":dbl[]}[])
        n109 = Replace Array Subset(array=w164, new element=w163, index=w154) -> (w162:cluster{"Duration":dbl[]}[])
        n110 = Replace Array Subset(array=w153, new element=w159, index=w154) -> (w157:cluster{"Duration":dbl[]}[])
        n111 = Bundle By Name(cluster=w176, "Local Data.Position Difference"=w157, "Local Data.Peak Velocity"=w156, "Local Data.Duration"=w162) -> (w175:cluster{"EMA-Data IN":T4, "Local Data":T7})
        n112 = Enqueue Element(queue=w186, element=w180) -> (queue out=w187:refnum<queue>)  [unwired: 2 in, 2 out]
      }
      frame "Display Main Sequence" {
        w262 = dbl[] []
        # "Fits a 2nd order polynom to the sum of datapoints (up to 4 amendments)"
        # "/\\ If Amend Box is active, this Variable is not  \n |  reseted to 0 and the next round will be amended \n |  to the present data."
        # "Unbundle Datapoints for up to 4\namendments and display them \nin individual colours"
        # "Calculates the mean Duration using all datapoints"
        # "Fits a 2nd order polynom to the sum of datapoints (up to 4 amendments)"
        n113 = Unbundle By Name(w261) -> ("Local Data.EYE"=w258:string[], "Local Data.Direction"=w257:bool[], "Local Data.Amendments"=w256:i32, "Local Data.Position Difference"=w276:cluster{"Duration":dbl[]}[], "Local Data.Peak Velocity"=w275:cluster{"Duration":dbl[]}[], "Local Data.Duration"=w279:cluster{"Duration":dbl[]}[], "EMA-Data IN.Data File.Sample Rate"=w278:i32)
        n114 = property on="Channel Position" class="Ring (strict)"() -> ("RingText.Text"=w252:string)  [unwired: 2 in, 2 out]
        n115 = for {
          tunnel: w279 -> [w301] mode=indexing
          tunnel: w278 -> [w300]
          tunnel: w276 -> [w299] mode=indexing
          tunnel: w275 -> [w298] mode=indexing
          tunnel: [w296] -> w270 mode=indexing
          shift-right: [w294] -> w236
          shift-left: w262 -> [w295]
          shift-right: [w292] -> w235
          shift-left: w262 -> [w293]
          shift-right: [w289] -> w239
          shift-left: w262 -> [w290]
          tunnel: [w287] -> w265 mode=indexing
          tunnel: [w286] -> w241 mode=indexing
          n116 = Unbundle(w299) -> ("Duration"=w288:dbl[])
          n117 = Unbundle(w298) -> ("Duration"=w291:dbl[])
          n118 = Unbundle(w301) -> ("Duration"=w297:dbl[])
          n119 = Divide(x=w297, y=w300) -> (x/y=w303:dbl[])
          n120 = Multiply(x=w303, y=1000) -> (x*y=w287:dbl[])
          n121 = Bundle("Duration"=w288, "Duration"=w291) -> (w296:cluster{"Duration":dbl[], "Duration":dbl[]})  [unwired: 1 in]
          n122 = Insert Into Array(array=w295, new element=w288) -> (w294:dbl[])  [unwired: 1 in]
          n123 = Insert Into Array(array=w293, new element=w291) -> (w292:dbl[])  [unwired: 1 in]
          n124 = Insert Into Array(array=w290, new element=w287) -> (w289:dbl[])  [unwired: 1 in]
          n125 = Bundle("Duration"=w288, w287) -> (w286:cluster{"Duration":dbl[], dbl[]})  [unwired: 1 in]
        }
        n126 = String Subset(string=w252, length (rest)=1 ("length (rest)")) -> (substring=w254:string)  [unwired: 1 in]
        n127 = case shown="\"R\"" w254 {
          tunnel: ["Unknown" "LEFT" "RIGHT"] -> w253
          frame "X", Default {
          }
          frame "L" {
          }
          frame "R" {
          }
        }
        n128 = local read "Direction"() -> (w251:bool)
        n129 = Build Array(w236, w239) -> (w243:dbl[][])
        n130 = Array Size(array=w265) -> (size(s)=w267:i32[])
        n131 = Build Array(w236, w235) -> (w273:dbl[][])
        n132 = call "Sort2D.vi"("2D array to sort"=w243) -> ("Sorted array"=w244:dbl[][])  [unwired: 4 in]
        n133 = call-poly <vilib>:"Mean.vi"("X"=w239) -> ("mean"=w248:dbl)  [unwired: 1 out]
        "Mean Saccade Duration [ms]" <- w248
        n134 = Array Max & Min(array=w267) -> (max value=w266:i32)  [unwired: 3 out]
        n135 = call "Sort2D.vi"("2D array to sort"=w273) -> ("Sorted array"=w272:dbl[][])  [unwired: 4 in]
        n136 = Replace Array Subset(array=w258, new element=w253, index=w256) -> (w249:string[])
        n137 = Replace Array Subset(array=w257, new element=w251, index=w256) -> (w250:bool[])
        n138 = Index Array(array=w244, index (col) #1=0 ("disabled index (col)")) -> (element #1=w238:dbl[], element #2=w240:dbl[])  [unwired: 3 in]
        n139 = Initialize Array(w248, w266) -> (w264:dbl[])
        n140 = Index Array(array=w272, index (col) #1=0 ("disabled index (col)")) -> (element #1=w232:dbl[], element #2=w233:dbl[])  [unwired: 3 in]
        n141 = Build Array (concatenate)(w265, w264) -> (→"Saccade Duration":dbl[][])
        n142 = call <vilib>:"General Polynomial Fit.vi"("Y"=w240, "polynomial order"=2, "X"=w238) -> ("Best Polynomial Fit"=w237:dbl[])  [unwired: 9 in, 3 out]
        n143 = call <vilib>:"General Polynomial Fit.vi"("Y"=w233, "polynomial order"=2, "X"=w232) -> ("Best Polynomial Fit"=w234:dbl[])  [unwired: 9 in, 3 out]
        n144 = Bundle("Sorted array"=w238, "Best Polynomial Fit"=w237) -> (w247:T9)  [unwired: 1 in]
        n145 = Bundle("Sorted array"=w232, "Best Polynomial Fit"=w234) -> (w268:T9)  [unwired: 1 in]
        n146 = Increment(x=w256) -> (x+1=w259:i32)
        n147 = Build Array (concatenate)(w241, w247) -> (→"Main Sequence - Duration vs Position":T10)
        n148 = Build Array (concatenate)(w270, w268) -> (→"Main Sequence - Velocity vs Position":T10)
        n149 = Bundle By Name(cluster=w261, "Local Data.EYE"=w249, "Local Data.Direction"=w250, "Local Data.Amendments"=w259) -> (w260:cluster{"EMA-Data IN":T4, "Local Data":T7})
        n150 = local write "Tab Control"(enum32{"Main Sequence", "Saccade Processing"}."Main Sequence" ("Tab Control")) -> ()
        n151 = Enqueue Element(queue=w281, element=cluster{string, "Variant":variant} {"Populate Table", "Variant"=variant}) -> (queue out=w282:refnum<queue>)  [unwired: 2 in, 2 out]
      }
      frame "Populate Table" {
        w310 = string[] []
        w323 = dbl[] []
        # "Unbundle Datapoints for up to 4\namendments and display them \nin individual colours"
        n152 = Unbundle By Name(w305) -> ("Local Data.EYE"=w318:string[], "Local Data.Direction"=w317:bool[], "Local Data.Position Difference"=w322:cluster{"Duration":dbl[]}[], "Local Data.Peak Velocity"=w321:cluster{"Duration":dbl[]}[], "Local Data.Duration"=w320:cluster{"Duration":dbl[]}[], "EMA-Data IN.Data File.Sample Rate"=w319:i32)
        n153 = for {
          tunnel: w320 -> [w353] mode=indexing
          tunnel: w319 -> [w352]
          tunnel: w322 -> [w351] mode=indexing
          tunnel: w321 -> [w350] mode=indexing
          shift-right: [w347] -> w307
          shift-left: w323 -> [w348]
          shift-right: [w345] -> w316
          shift-left: w323 -> [w346]
          shift-right: [w342] -> w315
          shift-left: w323 -> [w343]
          tunnel: [w340] -> _ mode=indexing
          tunnel: w318 -> [w339] mode=indexing
          tunnel: w317 -> [w341] mode=indexing
          shift-right: [w330] -> w308
          shift-left: w310 -> [w332]
          shift-right: [w331] -> w309
          shift-left: w310 -> [w333]
          n154 = Unbundle(w351) -> ("Duration"=w338:dbl[])
          n155 = Unbundle(w350) -> ("Duration"=w344:dbl[])
          n156 = Unbundle(w353) -> ("Duration"=w349:dbl[])
          n157 = case shown="False" w341 {
            tunnel: ["POS" "NEG"] -> w337
            frame True {
            }
            frame False {
            }
          }
          n158 = Divide(x=w349, y=w352) -> (x/y=w340:dbl[])
          n159 = Array Size(array=w338) -> (size(s)=w336:i32)
          n160 = Initialize Array(w337, w336) -> (w334:string[])
          n161 = Initialize Array(w339, w336) -> (w335:string[])
          n162 = Insert Into Array(array=w348, new element=w338) -> (w347:dbl[])  [unwired: 1 in]
          n163 = Insert Into Array(array=w346, new element=w344) -> (w345:dbl[])  [unwired: 1 in]
          n164 = Insert Into Array(array=w343, new element=w340) -> (w342:dbl[])  [unwired: 1 in]
          n165 = Insert Into Array(array=w333, new element=w334) -> (w331:string[])  [unwired: 1 in]
          n166 = Insert Into Array(array=w332, new element=w335) -> (w330:string[])  [unwired: 1 in]
        }
        n167 = Array Size(array=w307) -> (size(s)=w306:i32)
        n168 = Number To Fractional String(number=w307) -> (F-format string=w324:string[])  [unwired: 3 in]
        n169 = Number To Fractional String(number=w316) -> (F-format string=w313:string[])  [unwired: 3 in]
        n170 = Number To Fractional String(number=w315, precision (6)=i16 3) -> (F-format string=w312:string[])  [unwired: 2 in]
        n171 = Build Array(w309, w308, w324, w313, w312) -> (w311:string[][])
        n172 = Transpose 2D Array(2D array=w311) -> (transposed array=w325:string[][])
        n173 = local write "Table"(w325) -> ()
        n174 = Bundle By Name(cluster=w305, "Local Data.Table1 size"=w306) -> (w304:cluster{"EMA-Data IN":T4, "Local Data":T7})
        n175 = Enqueue Element(queue=w327, element=cluster{string, "Variant":variant} {"Idle", "Variant"=variant}) -> (queue out=w328:refnum<queue>, timed out?=w329:bool)  [unwired: 2 in, 1 out]
      }
      frame "Extract Features 1" {
        w381 = enum32{"Peaks", "Valleys"}."Valleys" ("peaks/valleys")
        # "Use the data before the Saccade Onset to calculate the Mean and Standard-Deviation of the Noise."
        # "Use either the valley of Acc or Vel  depending on which comes first"
        # "Check 20ms previous to Acc peak for a valley and uses it as Saccade onset"
        # "/\\ Find the highest acceleration\n |  peak and suspect that this is \n |  the saccade onset. \n |  (I know quite an assumption)"
        # "Disable Filter if neccessary"
        n176 = Unbundle By Name(w393) -> ("Local Data.Position"=w398:dbl[][], "Local Data.Velocity"=w397:dbl[][], "Local Data.Saccade Counter"=w396:i32, "EMA-Data IN.Data File.Sample Rate"=w380:i32)
        n177 = call "Time2Points.vi"("Time [ms]"=25.0, "Sample Rate"=w380) -> ("Points"=w386:i32)  [unwired: 2 in]
        n178 = call "Time2Points.vi"("Time [ms]"=25.0, "Sample Rate"=w380) -> ("Points"=w385:i32)  [unwired: 2 in]
        n179 = Index Array(array=w398, index (row)=w396) -> (element=w391:dbl[])  [unwired: 1 in]
        n180 = Index Array(array=w397, index (row)=w396) -> (element=w395:dbl[])  [unwired: 1 in]
        n181 = case shown="False" FALSE {
          tunnel: w395 -> [w473 w475]
          tunnel: [w473 w474] -> w372
          frame False {
          }
          frame True {
            n182 = call-poly <vilib>:"Savitzky-Golay Filter.vi"("polynomial order"=6, "side points"=4, "X"=w475) -> ("Filtered X"=w474:dbl[])  [unwired: 7 in, 1 out]
          }
        }
        n183 = call <vilib>:"Derivative x(t).vi"("X"=w372) -> ("dX/dt"=w375:dbl[])  [unwired: 9 in, 1 out]
        n184 = Array Max & Min(array=w375) -> (max index (indices)=w365:i32)  [unwired: 3 out]
        n185 = Subtract(x=w365, y=w386) -> (x-y=w388:i32)
        n186 = Subtract(x=w365, y=w385) -> (x-y=w368:i32)
        n187 = Array Subset(array=w372, length=w368) -> (w373:dbl[])  [unwired: 1 in]
        n188 = call <vilib>:"Std Deviation and Variance.vi"("X"=w373) -> ("mean"=w357:dbl, "standard deviation"=w356:dbl)  [unwired: 1 in, 1 out]
        n189 = Array Subset(array=w375, index=w368, length=w385) -> (w382:dbl[])
        n190 = Array Subset(array=w372, index=w388, length=w386) -> (w390:dbl[])
        n191 = Multiply(x=w356, y=2.5) -> (x*y=w371:dbl)
        n192 = Reverse 1D Array(array=w382) -> (reversed array=w383:dbl[])
        n193 = Reverse 1D Array(array=w390) -> (reversed array=w389:dbl[])
        n194 = Add(x=w357, y=w371) -> (x+y=w370:dbl)
        n195 = Subtract(x=w357, y=w371) -> (x-y=w366:dbl)
        n196 = call <vilib>:"Peak Detector.vi"("peaks/valleys"=w381, "X"=w389) -> ("Amplitudes"=w377:dbl[], "Locations"=w378:dbl[])  [unwired: 5 in, 3 out]
        n197 = call <vilib>:"Peak Detector.vi"("peaks/valleys"=w381, "threshold"=100.0, "X"=w383) -> ("Locations"=w376:dbl[])  [unwired: 4 in, 4 out]
        n198 = disable-structure shown="Enabled" {
          disable-tunnel: [w403 -inf] -> w367
          disable-tunnel: w366 -> [w403 _]
          frame Disabled {
          }
          frame Enabled {
          }
        }
        n199 = for {
          N: 3 -> [_]
          tunnel: w378 -> [w427]
          tunnel: w377 -> [w426]
          tunnel: w376 -> [w425]
          tunnel: w372 -> [w408]
          tunnel: w365 -> [w424]
          tunnel: w370 -> [w423]
          tunnel: w367 -> [w422]
          tunnel: [w414] -> w364
          tunnel: w368 -> [w407]
          tunnel: [w405] -> w358
          i -> [w413]
          stop <- w410 stop-if-true
          n200 = Index Array(array=w427, index=w413) -> (element=w429:dbl)
          n201 = Index Array(array=w426, index=w413) -> (element=w416:dbl)
          n202 = Index Array(array=w425, index=w413) -> (element=w428:dbl)
          n203 = Subtract(x=w424, y=w429) -> (x-y=w420:dbl)
          n204 = Subtract(x=w424, y=w428) -> (x-y=w419:dbl)
          n205 = Greater Or Equal?(x=w413, y=2) -> (x >= y?=w411:bool)
          n206 = Index Array(array=w408, index=w419) -> (element=w415:dbl)
          n207 = In Range and Coerce(upper limit=w423, x=w416, lower limit=w422) -> (In Range?=w418:bool)  [unwired: 1 out]
          n208 = In Range and Coerce(upper limit=w423, x=w415, lower limit=w422) -> (In Range?=w417:bool)  [unwired: 1 out]
          n209 = Or(x=w418, y=w417) -> (x .or. y?=w410:bool)
          n210 = Not(x=w410) -> (.not. x?=w406:bool)
          n211 = And(x=w418, y=w417) -> (x .and. y?=w421:bool)
          n212 = And(x=w406, y=w411) -> (x .and. y?=w409:bool)
          n213 = case shown="False" w421 {
            tunnel: w420 -> [w438 w463]
            tunnel: w419 -> [w436 w460]
            tunnel: w418 -> [w439 _]
            tunnel: w417 -> [_ _]
            tunnel: w416 -> [w437 w462]
            tunnel: w415 -> [w435 w459]
            tunnel: [w434 w461] -> w414
            tunnel: w409 -> [w433 _]
            tunnel: w408 -> [w432 _]
            tunnel: w407 -> [w431 _]
            tunnel: [w430 _] -> w405
            frame False {
              n214 = case shown="True" w433 {
                tunnel: w439 -> [w446 _]
                tunnel: w438 -> [w444 _]
                tunnel: w437 -> [w443 _]
                tunnel: w436 -> [w442 _]
                tunnel: w435 -> [w441 _]
                tunnel: [w440 w457] -> w434
                tunnel: w432 -> [_ w458]
                tunnel: w431 -> [_ w456]
                tunnel: [_ TRUE] -> w430
                frame False {
                  n215 = Not Equal To 0?(x=w444) -> (x != 0?=w447:bool)
                  n216 = And(x=w447, y=w446) -> (x .and. y?=w445:bool)
                  n217 = case shown="False" w445 {
                    tunnel: w444 -> [_ w453]
                    tunnel: w443 -> [_ w452]
                    tunnel: [w448 w451] -> w440
                    tunnel: w442 -> [w450 _]
                    tunnel: w441 -> [w449 _]
                    frame False {
                      n218 = Bundle(w450, "Numeric"=w449) -> (w448:cluster{dbl, "Numeric":dbl})  [unwired: 1 in]
                    }
                    frame True {
                      n219 = Bundle(w453, w452) -> (w451:cluster{dbl, dbl})  [unwired: 1 in]
                    }
                  }
                }
                frame True {
                  n220 = Index Array(array=w458, index=w456) -> (element=w455:dbl)
                  n221 = Bundle(w456, "Numeric"=w455) -> (w457:cluster{i32, "Numeric":dbl})  [unwired: 1 in]
                }
              }
            }
            frame True {
              n222 = Not Equal To 0?(x=w463) -> (x != 0?=w465:bool)
              n223 = Greater?(x=w463, y=w460) -> (0:w466:bool)
              n224 = And(x=w465, y=w466) -> (x .and. y?=w464:bool)
              n225 = case shown="False" w464 {
                tunnel: w463 -> [_ w472]
                tunnel: w462 -> [_ w471]
                tunnel: [w467 w470] -> w461
                tunnel: w460 -> [w469 _]
                tunnel: w459 -> [w468 _]
                frame False {
                  n226 = Bundle(w469, "Numeric"=w468) -> (w467:cluster{dbl, "Numeric":dbl})  [unwired: 1 in]
                }
                frame True {
                  n227 = Bundle(w472, w471) -> (w470:cluster{dbl, dbl})  [unwired: 1 in]
                }
              }
            }
          }
        }
        n228 = Unbundle(w364) -> (w360:dbl, "Numeric"=w359:dbl)
        n229 = Bundle By Name(cluster=w393, "Local Data.Single Position"=w391, "Local Data.Single Velocity"=w372, "Local Data.Single Acceleration"=w375, "Local Data.Saccade Onset"=w364, "Local Data.Acceleration Peak"=w365, "Local Data.Mean Noise"=w357, "Local Data.SD Noise"=w356) -> (w392:cluster{"EMA-Data IN":T4, "Local Data":T7})
        n230 = Not A Number/Path/Refnum?(number/path/refnum=w360) -> (NaN/Path/Refnum?=w363:bool)
        n231 = Not A Number/Path/Refnum?(number/path/refnum=w359) -> (NaN/Path/Refnum?=w362:bool)
        n232 = Compound Arithmetic op=OR(w363, w362, w358) -> (w361:bool)
        n233 = local write "Skip for Analysis"(w361) -> ()
        n234 = Enqueue Element(queue=w400, element=cluster{string, "Variant":variant} {"Extract Features 2", "Variant"=variant}) -> (queue out=w401:refnum<queue>)  [unwired: 2 in, 2 out]
      }
      frame "Extract Features 2" {
        # "Mean of the Noisy Data after \napproximated Saccade End to use for intercept"
        # "5. Find the intercept with the \nMean of the acceleration data noise (which seams to be more stable than mean of velocity)"
        # "4. Line fit to the descending part of the Velocity data. \nSubsequently the line fit is masked with NaN so that the \nfit is only visible in the  descending part when plotted."
        # "3. Make Mask for Line-fit"
        # "2. Look for the first Peak after the last Valley. This Peak is close to the endo of the saccade. \nIt is used as the End-Point for the Line fit"
        # "1. Look for Valleys that occur 50ms after the velocity peak, and exeed 4xSD of Noise"
        n235 = Unbundle By Name(w524) -> ("Local Data.Single Velocity"=w489:dbl[], "Local Data.Single Acceleration"=w490:dbl[], "EMA-Data IN.Data File.Sample Rate"=w496:i32, "Local Data.Saccade Onset.X"=w491:dbl, "Local Data.Acceleration Peak"=w488:i32)
        n236 = call "Time2Points.vi"("Time [ms]"=70.0, "Sample Rate"=w496) -> ("Points"=w520:i32)  [unwired: 2 in]
        n237 = disable-structure shown="Enabled" {
          disable-tunnel: [w534 0.0 ("threshold")] -> w519
          disable-tunnel: w490 -> [w532 _]
          disable-tunnel: w491 -> [w531 _]
          frame Enabled {
            # "Use the data before the Saccade Onset to calculate the Mean and Standard-Deviation of the Noise."
            n238 = Array Subset(array=w532, length=w531) -> (w539:dbl[])  [unwired: 1 in]
            n239 = call <vilib>:"Std Deviation and Variance.vi"("X"=w539) -> ("mean"=w533:dbl, "standard deviation"=w538:dbl)  [unwired: 1 in, 1 out]
            n240 = Multiply(x=w538, y=3.0) -> (x*y=w536:dbl)
            n241 = Negate(x=w536) -> (-x=w535:dbl)
            n242 = Add(x=w533, y=w535) -> (x+y=w534:dbl)
          }
          frame Disabled {
          }
        }
        n243 = Array Subset(array=w490, index=w488, length=w520) -> (w517:dbl[])
        n244 = call <vilib>:"Peak Detector.vi"("peaks/valleys"=enum32{"Peaks", "Valleys"}."Valleys", "threshold"=w519, "X"=w517) -> ("Locations"=w518:dbl[])  [unwired: 4 in, 4 out]
        n245 = Array Max & Min(array=w518) -> (max value=w508:dbl)  [unwired: 3 out]
        n246 = Add(x=w488, y=w508) -> (x+y=w507:dbl)
        n247 = call "Time2Points.vi"("Time [ms]"=30.0, "Sample Rate"=w496) -> ("Points"=w516:i32)  [unwired: 2 in]
        n248 = Array Subset(array=w490, index=w507, length=w516) -> (w514:dbl[])
        n249 = call <vilib>:"Peak Detector.vi"("peaks/valleys"=enum32{"Peaks", "Valleys"}."Peaks", "X"=w514) -> ("Locations"=w486:dbl[])  [unwired: 5 in, 4 out]
        n250 = Index Array(array=w486) -> (element=w484:dbl)  [unwired: 1 in]
        n251 = Empty Array?(array=w486) -> (empty?=w487:bool)
        n252 = case shown="True" w487 {
          tunnel: [w529 1] -> w485
          tunnel: w484 -> [w529 _]
          frame False {
          }
          frame True {
          }
        }
        n253 = Add(x=w507, y=w485) -> (x+y=w492:dbl)
        n254 = Array Size(array=w489) -> (size(s)=w494:i32)
        n255 = Subtract(x=w494, y=w492) -> (x-y=w495:dbl)
        n256 = Array Subset(array=w489, index=w492, length=w495) -> (w493:dbl[])
        n257 = call <vilib>:"Std Deviation and Variance.vi"("X"=w493) -> ("mean"=w482:dbl)  [unwired: 1 in, 2 out]
        n258 = Array Max & Min(array=w489) -> (max index (indices)=w501:i32)  [unwired: 3 out]
        n259 = Subtract(x=w492, y=w501) -> (x-y=w498:dbl)
        n260 = Increment(x=w498) -> (x+1=w497:dbl)
        n261 = Initialize Array(0.0 ("element"), w494) -> (w511:dbl[])
        n262 = call-poly <vilib>:"Ramp Pattern.vi"("end"=w494, "samples"=w494) -> ("Ramp Pattern"=w506:dbl[])  [unwired: 8 in, 1 out]
        n263 = Initialize Array(1.0 ("element"), w497) -> (w509:dbl[])
        n264 = Negate(x=w482) -> (-x=w499:dbl)
        n265 = Replace Array Subset(array=w511, new element=w509, index=w501) -> (w504:dbl[])
        n266 = local read "Skip for Analysis"() -> (w478:bool)
        n267 = call <vilib>:"Linear Fit.vi"("Y"=w489, "X"=w506, "Weight"=w504) -> ("Best Linear Fit"=w503:dbl[])  [unwired: 8 in, 4 out]
        n268 = Negate(x=w503) -> (-x=w500:dbl[])
        n269 = Threshold 1D Array(1:w501, 2:w499, 3:w500) -> (0:w483:dbl)
        n270 = call "Mask with NaN.vi"("Mask"=w504, "Array IN"=w503) -> ("Array OUT"=w505:dbl[])  [unwired: 2 in]
        n271 = Not A Number/Path/Refnum?(number/path/refnum=w483) -> (NaN/Path/Refnum?=w481:bool)
        n272 = Not A Number/Path/Refnum?(number/path/refnum=w482) -> (NaN/Path/Refnum?=w480:bool)
        n273 = Bundle(w483, "mean"=w482) -> (w502:cluster{dbl, "mean":dbl})  [unwired: 1 in]
        n274 = Bundle By Name(cluster=w524, "Local Data.Linear Fit"=w505, "Local Data.Saccade End"=w502) -> (w523:cluster{"EMA-Data IN":T4, "Local Data":T7})
        n275 = Compound Arithmetic op=OR(w481, w480, w478) -> (w479:bool)
        n276 = local write "Skip for Analysis"(w479) -> ()
        n277 = Enqueue Element(queue=w526, element=cluster{string, "Variant":variant} {"Display Single Saccade", "Variant"=variant}) -> (queue out=w527:refnum<queue>)  [unwired: 2 in, 2 out]
      }
      frame "Display Single Saccade" {
        # "Lets the Pause Button flash to make the user aware of the pressed Pause button"
        # "If the pause button is active --> go to \nIdle and wait there until the next button \nor Skip-Forward Button is pressed"
        # "Saccade Onset and End Point"
        # "Calculate Time Array"
        n278 = local read "Tab Control"() -> (w544:T1)
        n279 = Unbundle By Name(w573) -> ("EMA-Data IN.Data File.Sample Rate"=w571:i32, "Local Data.Single Velocity"=w570:dbl[], "Local Data.Single Acceleration"=w568:dbl[], "Local Data.Saccade Onset"=w566:cluster{"X":dbl, "Y":dbl}, "Local Data.Linear Fit"=w554:dbl[], "Local Data.Saccade End"=w553:cluster{"X":dbl, "Y":dbl}, "Local Data.Mean Noise"=→"Mean Noise":dbl, "Local Data.SD Noise"=→"SD Noise":dbl)
        n280 = Not Equal?(x=enum32{"Main Sequence", "Saccade Processing"}."Saccade Processing" ("Tab Control"), y=w544) -> (x != y?=w543:bool)
        n281 = Compound Arithmetic op=AND(w543, "Pause Button") -> (w547:bool)
        n282 = case shown="True" w547 {
          frame False {
          }
          frame True {
            n283 = flat-sequence {
              frame #0 {
                n284 = local write "Tab Control"(enum32{"Main Sequence", "Saccade Processing"}."Saccade Processing" ("Tab Control")) -> ()
              }
              frame #1 {
                n285 = for {
                  N: 5 -> [_]
                  n286 = flat-sequence {
                    frame #0 {
                      n287 = Wait (ms)(milliseconds to wait=u32 180) -> ()  [unwired: 1 out]
                    }
                    frame #1 {
                      n288 = property on="Pause Button" class="Bool (strict)"("Value"=FALSE ("Pause Button")) -> ()  [unwired: 2 in, 2 out]
                    }
                    frame #2 {
                      n289 = Wait (ms)(milliseconds to wait=u32 180) -> ()  [unwired: 1 out]
                    }
                    frame #3 {
                      n290 = property on="Pause Button" class="Bool (strict)"("Value"=TRUE ("Pause Button")) -> ()  [unwired: 2 in, 2 out]
                    }
                  }
                }
              }
            }
          }
        }
        n291 = Reciprocal(x=w571) -> (1/x=w563:dbl)
        n292 = Unbundle(w553) -> ("X"=w552:dbl, "Y"=w551:dbl)
        n293 = Unbundle(w566) -> ("X"=w561:dbl, "Y"=w559:dbl)
        n294 = Array Size(array=w570) -> (size(s)=w562:i32)
        n295 = call-poly <vilib>:"Ramp Pattern.vi"("end"=w562, "samples"=w562) -> ("Ramp Pattern"=w572:dbl[])  [unwired: 8 in, 1 out]
        n296 = Build Array(w561, w552) -> (w560:dbl[])
        n297 = Build Array(w559, w551) -> (w558:dbl[])
        n298 = Multiply(x=w572, y=w563) -> (x*y=w555:dbl[])
        n299 = Multiply(x=w560, y=w563) -> (x*y=w557:dbl[])
        n300 = Bundle(w555, "Linear Fit"=w554) -> (w556:cluster{dbl[], "Linear Fit":dbl[]})  [unwired: 1 in]
        n301 = Bundle(w555, "Single Velocity"=w570) -> (w569:cluster{dbl[], "Single Velocity":dbl[]})  [unwired: 1 in]
        n302 = Bundle(w555, "Single Acceleration"=w568) -> (w567:cluster{dbl[], "Single Acceleration":dbl[]})  [unwired: 1 in]
        n303 = Bundle(w557, w558) -> (w565:cluster{dbl[], dbl[]})  [unwired: 1 in]
        n304 = Build Array(w569, w567, w565, w556) -> (→"Single Saccade Display":cluster{dbl[], "Linear Fit":dbl[]}[])
        n305 = Select(t=cluster{string, "Variant":variant} {"Idle", "Variant"=variant} ("element"), s="Pause Button", f=cluster{string, "Variant":variant} {"Next Saccade", "Variant"=variant} ("element")) -> (s? t:f=w548:cluster{string, "Variant":variant})
        n306 = Enqueue Element(queue=w574, element=w548) -> (queue out=w575:refnum<queue>)  [unwired: 2 in, 2 out]
      }
      frame "Get Saccades" {
        # "If the data should be overwritten, the variable \"Amendments\" is reseted. Otherwise only \"Saccade Count\" is reseted"
        # "Inverts the signal if\nthe tallest peak is to \nthe negative side"
        # "Saccades that go to the negative side\nare inverted to make the analysis \neasier."
        # "List to extract Position and Velocity"
        n307 = Unbundle By Name(w586) -> ("Local Data.Direction Plot"=w583:bool)
        n308 = Unbundle By Name(w586) -> ("EMA-Data IN.Data File"=w610:T11, "EMA-Data IN.Impulse Positions"=w609:T12, "EMA-Data IN.desaccading parameters.Impulse Plane 2"=w608:T13, "EMA-Data IN.Parameter Impuls Series"=w605:T6)
        n309 = local read "Channel Position"() -> (w602:u16)
        n310 = local read "Channel Velocity"() -> (w601:u16)
        n311 = Index Array(array=w605) -> (element=w606:T14)  [unwired: 1 in]
        n312 = Initialize Array(w606, 2 ("dimension size")) -> (w603:T15)
        n313 = Build Array(w602, w601) -> (w604:u16[])
        n314 = for {
          tunnel: w603 -> [w637] mode=indexing
          tunnel: [w636] -> w600 mode=indexing
          tunnel: w604 -> [w635] mode=indexing
          n315 = Bundle By Name(cluster=w637, "Channel"=w635) -> (w636:T14)
        }
        n316 = call "Couple Head Impulse Traces.vi"("Data Input"=w610, "Impulse Positions"=w609, "Impulse Direction +ve?"=w583, "Impulse Plane"=w608, "Plot Selection 2"=w600) -> ("No Impulses"=w598:i32, "Impulses"=w599:dbl[][])  [unwired: 11 in, 2 out]
        n317 = case shown="False" "Amend" {
          tunnel: w586 -> [w616 w627]
          tunnel: [w615 w626] -> w585
          frame True {
            n318 = Bundle By Name(cluster=w616, "Local Data.Saccade Counter"=0) -> (w615:cluster{"EMA-Data IN":T4, "Local Data":T7})
          }
          frame False {
            w621 = 4 ("dimension size")
            n319 = Initialize Array(cluster{"Duration":dbl[]} {"Duration"=[]} ("Cluster"), w621) -> (w623:cluster{"Duration":dbl[]}[])
            n320 = Initialize Array("", w621) -> (w618:string[])
            n321 = Initialize Array(FALSE, w621) -> (w619:bool[])
            n322 = Bundle By Name(cluster=w627, "Local Data.Saccade Counter"=0, "Local Data.Position Difference"=w623, "Local Data.Peak Velocity"=w623, "Local Data.Duration"=w623, "Local Data.Amendments"=0, "Local Data.EYE"=w618, "Local Data.Direction"=w619) -> (w626:cluster{"EMA-Data IN":T4, "Local Data":T7})
          }
        }
        n323 = Array Subset(array=w599, length (row)=w598) -> (w588:dbl[][])  [unwired: 3 in]
        n324 = Array Subset(array=w599, index (row)=w598) -> (w594:dbl[][])  [unwired: 3 in]
        "Saccade Velocity" <- w594
        n325 = Array Max & Min(array=w594) -> (max value=w593:dbl, min value=w592:dbl)  [unwired: 2 out]
        n326 = Absolute Value(x=w593) -> (abs(x)=w591:dbl)
        n327 = Absolute Value(x=w592) -> (abs(x)=w590:dbl)
        n328 = Greater Or Equal?(x=w591, y=w590) -> (x >= y?=w589:bool)
        n329 = call "Fick to RV in 1 plane.vi"("Fick IN"=w588) -> ("Angle OUT"=w587:dbl[][])  [unwired: 4 in]
        "Saccade Position" <- w587
        n330 = case shown="False" w589 {
          tunnel: [w632 w634] -> w596
          tunnel: w587 -> [w631 w634]
          tunnel: [w629 w633] -> w595
          tunnel: w594 -> [w630 w633]
          frame False {
            n331 = Negate(x=w631) -> (-x=w632:dbl[][])
            n332 = Negate(x=w630) -> (-x=w629:dbl[][])
          }
          frame True {
          }
        }
        n333 = Bundle By Name(cluster=w585, "Local Data.Position"=w596, "Local Data.Velocity"=w595) -> (w597:cluster{"EMA-Data IN":T4, "Local Data":T7})
        n334 = Enqueue Element(queue=w612, element=cluster{string, "Variant":variant} {"Extract Features 1", "Variant"=variant}) -> (queue out=w613:refnum<queue>)  [unwired: 2 in, 2 out]
      }
    }
  }
  n335 = Flush Queue(queue=w4) -> (queue out=w6:refnum<queue>, error out=w5:errorcluster)  [unwired: 1 in, 1 out]
  n336 = Release Queue(queue=w6, error in (no error)=w5) -> ()  [unwired: 1 in, 3 out]
